vi "S4GEI.vi"() -> ()   [LabVIEW 2018]
uses:
  S4GEI/S4GEI.lvclass
  S4GEI/S4GEI.lvclass/S4GEI.ctl
  Channel GUI/Channel.lvclass/Channel.ctl
  Channel GUI/Channel.lvclass
  Camera/Camera.lvclass
  S4ICS/S4ICS.lvclass
  Mechanism/Mechanism.lvclass
panel:
  in  "Tab Control 2":T1(tab)
  in  "Stop Application":bool
  out "pol mode":bool
  out "phot mode":bool
  out "Error Message":string
  in  "wppos presents":u16(ring) items=["Clear", "All positions", "First 8 positions", "First 4 positions", "1-4 & 9-12", "Customized"]
  in  "waveplate":u16(ring)=2 items=["OFF"=2, "L/2"=3, "L/4"=1]
  in  "calib wheel":u16(ring)=3 items=["OFF"=3, "PINHOLE"=1, "POLARIZER"=2, "SHUTTER"=4, "DEPOLARIZER"=5]
  in  "waveplate positions":T2={"WP 1"=TRUE, "WP 2"=FALSE, "WP 3"=FALSE, "WP 4"=FALSE, "WP 5"=FALSE, "WP 6"=FALSE, "WP 7"=FALSE, "WP 8"=FALSE, "WP 9"=FALSE, "WP 10"=FALSE, "WP 11"=FALSE, "WP 12"=FALSE, "WP 13"=FALSE, "WP 14"=FALSE, "WP 15"=FALSE, "WP 16"=FALSE}
  out "current calw":u16(ring)=3 items=["PINHOLE"=1, "POLARIZER"=2, "OFF"=3, "SHUTTER"=4, "DEPOLARIZER"=5]
  out "current waveplate":u16(ring)=2 items=["L/4"=1, "OFF"=2, "L/2"=3]
  out "analyser status":bool
  out "current wppos":T2
  in  "start exp":bool
  in  "Stop Acquisition":bool
  in  "Abort Acquisition":bool
  in  "Pause acquisition":bool
  in  "exp time":dbl=1.5 min=9.999999747378752e-06
  in  "#frames":u16=1 min=1 max=1000
  in  "#cycles":u32=1 min=1
  in  "Send Message":bool
  in  "Command:":string
  in  "FWCS IP":string="200.131.64.49"
  in  "ACS IP":string="200.131.64.25"
  in  "Channel ID":u16=1 min=1
  out "CCD status":T3={"Cycles done"=1, "Sequences done"=1, "Frames done"=1, "CCD Status"="", "Exposing"=FALSE, "Last image"="", "temp"=0, "serial n"=0, "texp"=0.0, "used disk"=0, "power"=FALSE, "acs mode"=FALSE} {"Frames done" max=2 scale=0.0..1.0; "Sequences done" max=8 scale=0.0..1.0; "Cycles done" max=2 scale=0.0..1.0}
  in  "projid":string="ENG"
  in  "observer":string="Denis"
  in  "object name":string="Test"
  in  "comment":string
  in  "file name suffix":string
  in  "preset modes":T4
  in  "auto adv mode":bool
  in  "Cooler":bool
  in  "Temp":i32=20 min=-80 max=20
  in  "Set camera configuration":bool
  in  "EM Gain":u16=2
  in  "EM Mode":u8(ring)=1 items=["Electron Multiplying", "Conventional", "Error"]
  in  "Readout Rate":u8(ring) items=["1 MHz", "0.1 MHz"]
  in  "Pre-amp gain":u8(ring) items=["Gain 1", "Gain 2", "Error"]
  in  "Vertical Clock Voltagem":u16(ring) items=["Normal", "+1", "+2", "+3", "+4", "Error"]
  in  "Acquisition Mode":u16(ring)=3 items=["Reserved", "Single Scan", "Accumulate", "Kinetic", "Fast Kinetic", "Run till abort", "Reserved", "Reserved", "Reserved", "Time Delayed Integration"]
  in  "Read Mode":u16(ring)=4 items=["Full Vertical Binning", "Multi-Track", "Random-Track", "Single-Track", "Image"]
  in  "Trigger Mode":u16(ring) items=["Internal", "External", "N/A", "N/A", "N/A", "N/A", "External Start", "External Exposure (Bulb)", "N/A", "External FVB EM", "Software", "N/A", "External Charge Shifting"]
  in  "Vertical Shift Speed":u16(ring)=3 items=["0.6", "1.13", "2.2", "4.33", "Error"]
  in  "AD Channel":u16
  in  "Shutter Mode":u8(ring)=2 items=["OPEN"=1, "CLOSED"=2, "Error"=3]
  in  "Shutter Time":u16=50
  in  "Shutter TTL":u16(ring) items=["TTL Low", "TTL High", "Error"]
  in  "Binning":u16=1
  in  "Initial Line":u16=1
  in  "Initial Cloumn":u16=1
  in  "Final Column":u16=1024
  in  "Final Line":u16=1024
  in  "Sub Image":T5(radio)=enum."1024 x 1024"
  in  "Frame Tansfer":bool=TRUE
  in  "stop iterations":bool
  out "Exposing 2":bool
  out "Frame exp time (s) \n2":dbl
  out "Exposições realizadas 2":u16(slide)=1 max=2 scale=-1.0..1.0
  in  "Acquisition configuration 6":T6={"Select"=FALSE, "Exp Time"=1.0, "#Frames"=1, "Sufix"="", "Filter"=6} {"Filter" items=["U"=1, "B"=2, "V"=3, "R"=4, "I"=5, "Clear"=6]}
  in  "Acquisition configuration 5":T6={"Select"=FALSE, "Exp Time"=1.0, "#Frames"=1, "Sufix"="", "Filter"=5} {"Filter" items=["U"=1, "B"=2, "V"=3, "R"=4, "I"=5, "Clear"=6]}
  in  "Acquisition configuration 4":T6={"Select"=FALSE, "Exp Time"=1.0, "#Frames"=1, "Sufix"="", "Filter"=4} {"Filter" items=["U"=1, "B"=2, "V"=3, "R"=4, "I"=5, "Clear"=6]}
  in  "Acquisition configuration 3":T6={"Select"=FALSE, "Exp Time"=1.0, "#Frames"=1, "Sufix"="", "Filter"=3} {"Filter" items=["U"=1, "B"=2, "V"=3, "R"=4, "I"=5, "Clear"=6]}
  in  "Acquisition configuration 2":T6={"Select"=FALSE, "Exp Time"=1.0, "#Frames"=1, "Sufix"="", "Filter"=2} {"Filter" items=["U"=1, "B"=2, "V"=3, "R"=4, "I"=5, "Clear"=6]}
  in  "Number of iterations":u16=1
  out "Current filter":u16(ring)=1 items=["U"=1, "B"=2, "V"=3, "R"=4, "I"=5, "Clear"=6]
  in  "Start Iterations":bool
  out "Iterations Done":u16(slide) scale=0.0..1.0
  in  "Acquisition configuration":T6={"Select"=FALSE, "Exp Time"=1.0, "#Frames"=1, "Sufix"="", "Filter"=1} {"Filter" items=["U"=1, "B"=2, "V"=3, "R"=4, "I"=5, "Clear"=6]}
  out "WPROT status":T7
  out "WPSEL status":T7
  out "CALW status":T7
  out "ASEL status":T7
  out "GMIR status":T7
  out "GFOC status":T7
  # "Instrument mode:"
  # "SPARC4\nGraphical Engineering Interface (S4GEI)"
  # "AUTOMATIC ADVANCE MODE"
  # "FWCS Iterator"
  # "Select"
  # "Filter"
  # "#Frames"
  # "Exp time (s)"
  # "Suffix"
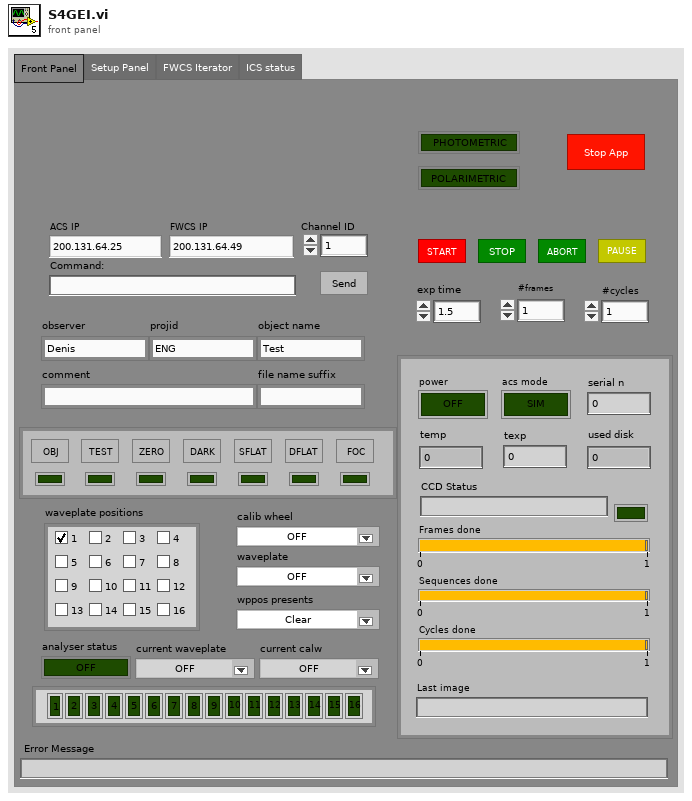
[diagram p1: front panel]
types:
  T1 = enum32{"Front Panel", "Setup Panel", "FWCS Iterator", "ICS status"}
  T2 = cluster{"WP 1":bool, "WP 2":bool, "WP 3":bool, "WP 4":bool, "WP 5":bool, "WP 6":bool, "WP 7":bool, "WP 8":bool, "WP 9":bool, "WP 10":bool, "WP 11":bool, "WP 12":bool, "WP 13":bool, "WP 14":bool, "WP 15":bool, "WP 16":bool}
  T3 = cluster{"Cycles done":u16, "Sequences done":u16, "Frames done":u16, "CCD Status":string, "Exposing":bool, "Last image":string, "temp":i16, "serial n":u16, "texp":dbl, "used disk":i16, "power":bool, "acs mode":bool}
  T4 = cluster{"OBJECT":bool, "TEST":bool, "ZERO":bool, "DARK":bool, "SFLAT":bool, "DFLAT":bool, "FOCUS":bool, "led object":bool, "led test":bool, "led zero":bool, "led dark":bool, "led sflat":bool, "led dflat":bool, "led foc":bool}
  T5 = enum32{"256 x 256", "512 x 512", "1024 x 1024", "Custom"}
  T6 = cluster{"Select":bool, "Exp Time":dbl, "#Frames":u16, "Sufix":string, "Filter":u16}
  T7 = cluster{"mode":string, "condition":string, "position":string, "pos_name":string, "pos_id":string}
  T8 = cluster{"FWCS IP":string, "ACS IP":string, "Channel ID":u16}
  T9 = enum8{"Enabled", "Disabled", "Disabled and Grayed Out"}
  T10 = cluster{"object":bool, "test":bool, "zero":bool, "dark":bool, "sflat":bool, "dflat":bool, "focus":bool, "object 2":bool, "test 2":bool, "zero 2":bool, "dark 2":bool, "sflat 2":bool, "dflat 2":bool, "foc":bool}
  T11 = cluster{"WP 1":bool, "WP 2":bool, "WP 3":bool, "WP 4":bool, "WP 5":bool, "WP 6":bool, "WP 9":bool, "WP 8":bool, "WP 7":bool, "WP 10":bool, "WP 11":bool, "WP 12":bool, "WP 13":bool, "WP 14":bool, "WP 15":bool, "WP 16":bool}
  T12 = cluster{"OBJECT":bool, "TEST":bool, "ZERO":bool, "DARK":bool, "SFLAT":bool, "DFLAT":bool, "FOCUS":bool}
  T13 = cluster{"CYCLES_DONE":u16, "LAST_IMAGE_NAME":string, "USED_DISK_SPACE":u16, "FRAMES_DONE":u16, "CCD_STATUS":string, "CURRENT_TEMPERATURE":i16, "TEMPERATURE_STATUS":string, "FRAME_EXPOSURE_TIME":sgl, "ERROR":bool, "SERIAL_NUMBER":u16, "ACQUIRING":bool, "IMAGE_INDEX":u32, "SEQS_DONE":u16, "POWER":bool, "ACS MODE":bool}
  T14 = cluster{"EXPTIME":dbl, "#FRAMES":u32, "#CYCLES":u32, "#SEQS":u32, "WAVEPLATE_POS":u16, "suffix":string, "TEMP":i32, "COOLER_POWER_STATUS":u16}
  T15 = cluster{"WPROT":refnum<class "Mechanism.lvclass">, "WPSEL":refnum<class "Mechanism.lvclass">, "CALW":refnum<class "Mechanism.lvclass">, "ASEL":refnum<class "Mechanism.lvclass">, "GMIR":refnum<class "Mechanism.lvclass">, "GFOC":refnum<class "Mechanism.lvclass">, "State Machine.lvclass":refnum<class "State Machine.lvclass">, "Status RxTx.lvclass":refnum<class "RxTx.lvclass">}
  T16 = cluster{"PREAMP":u16, "READOUT_RATE":u16, "EM_GAIN":u16, "VERTICAL_SHIFT_SPEED":u16, "READ_MODE":u16, "FRAME_TRANSFER":bool, "VERTICAL_CLOCK_VOLTAGE":u16, "ACQUISITION_MODE":u16, "AD_CHANNEL":u16, "EM_MODE":u16, "SHUTTER_TTL":u16, "SHUTTER_OPENING_TIME":u16, "SHUTTER_CLOSING_TIME":u16, "SHUTTER_MODE":u16, "TRIGGER_MODE":u16, "VBIN":u16, "INITIAL_LINE":u16, "INITIAL_COLUMN":u16, "FINAL_LINE":u16, "FINAL_COLUMN":u16, "HBIN":u16}
  T17 = cluster{"waveplate positions":cluster{"WP 1":bool, "WP 2":bool, "WP 3":bool, "WP 4":bool, "WP 5":bool, "WP 6":bool, "WP 9":bool, "WP 8":bool, "WP 7":bool, "WP 10":bool, "WP 11":bool, "WP 12":bool, "WP 13":bool, "WP 14":bool, "WP 15":bool, "WP 16":bool}, "wppos presents":u16, "calib wheel":u16, "waveplate":u16}
  T18 = cluster{"Acquire":bool, "Stop Acquisition":bool, "Abort Acquisition":bool, "Pause acquisition":bool}
  T19 = cluster{"OBJECT":string, "OBSERVER":string, "CTRLINTE":string, "PROJID":string, "SYNCMODE":string, "INSTMODE":string, "FILTER":string, "OBSTYPE":string, "GUIVRSN":string, "COMMENT":string, "broker":string, "timestamp":string, "CHANNEL 1":bool, "CHANNEL 2":bool, "CHANNEL 3":bool, "CHANNEL 4":bool, "TCSMODE":bool}
  T20 = cluster{"Cycles done":u16, "Sequences done":u16, "Frames done":u16, "CCD Status":string, "Exposing":bool, "Last image":string, "temp":i16, "serial n":u16, "texp":dbl, "used disk":i16, "Power":bool, "ACS mode":bool}
  T21 = cluster{"object":bool, "test":bool, "zero":bool, "dark":bool, "sflat":bool, "dflat":bool, "focus":bool, "led object":bool, "led test":bool, "led zero":bool, "led dark":bool, "led sflat":bool, "led dflat":bool, "led foc":bool}
  T22 = cluster{"Select":bool, "Exp Time":u16, "#Frames":u16, "Sufix":string, "Filter":u16}
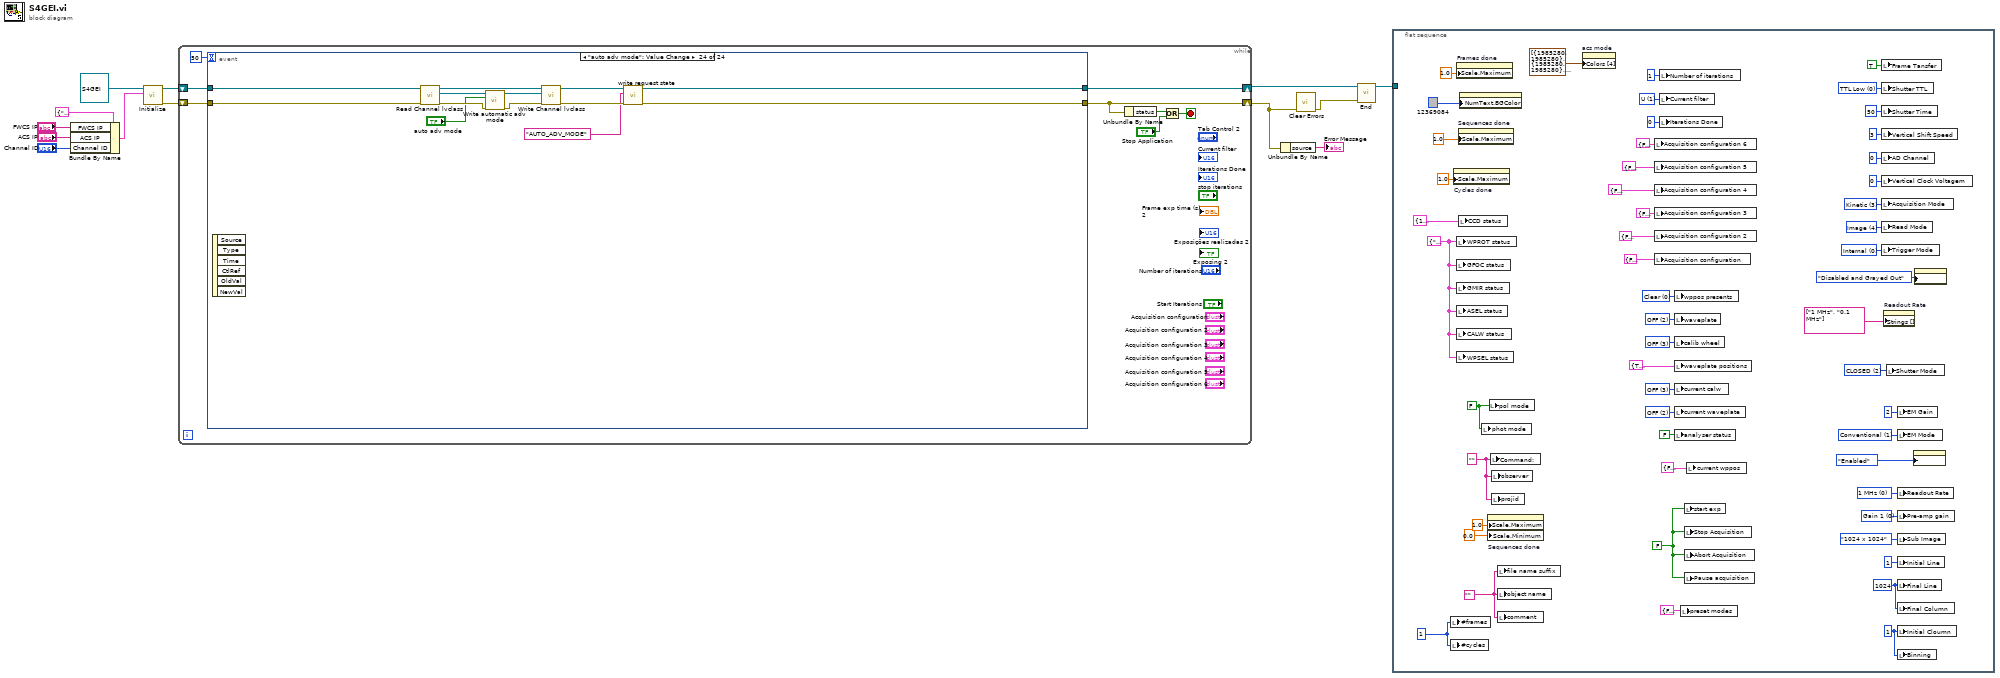
[diagram p0: block diagram]
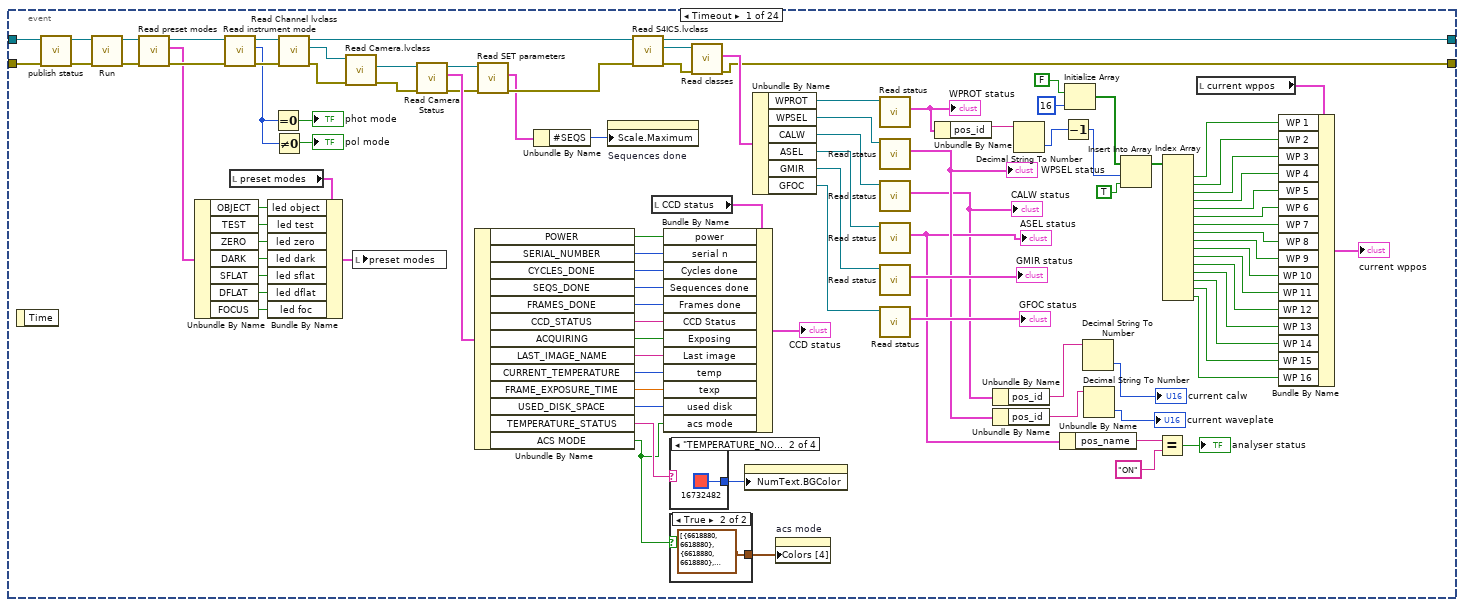
[diagram p2: hidden frame]
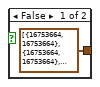
[diagram p3: hidden frame]
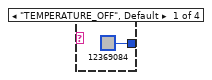
[diagram p4: hidden frame]
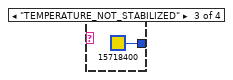
[diagram p5: hidden frame]
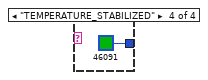
[diagram p6: hidden frame]
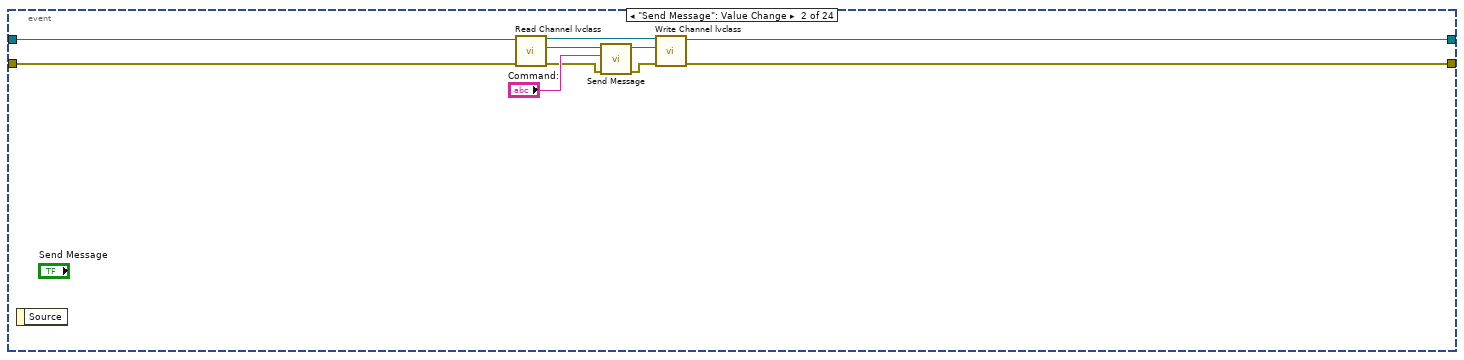
[diagram p7: hidden frame]
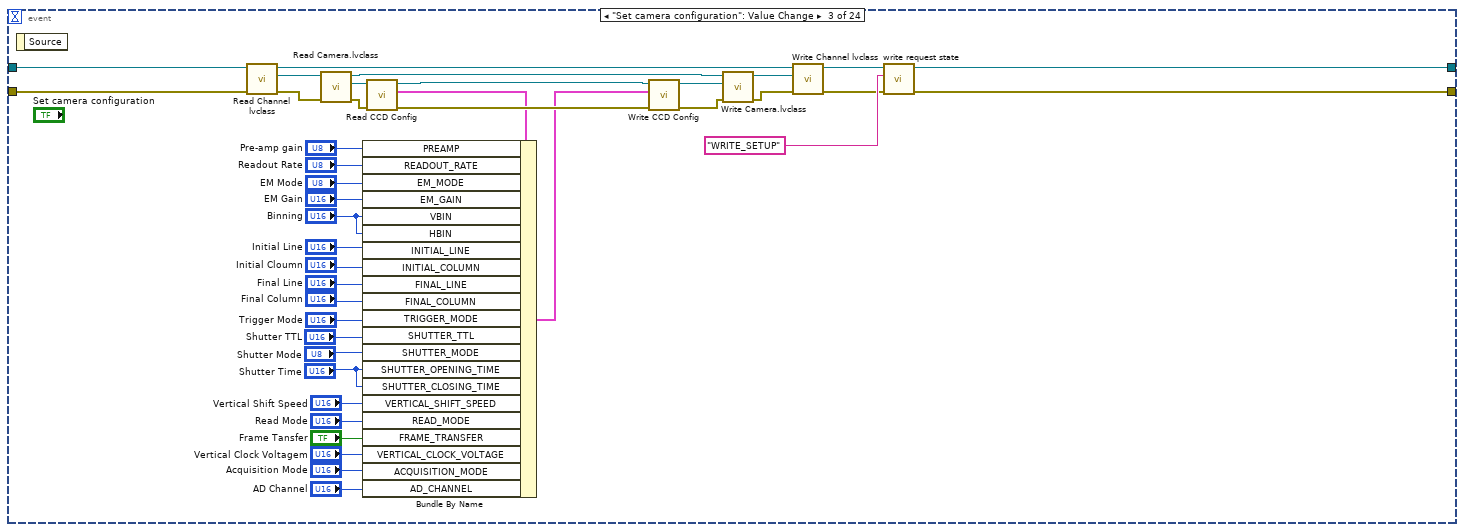
[diagram p8: hidden frame]
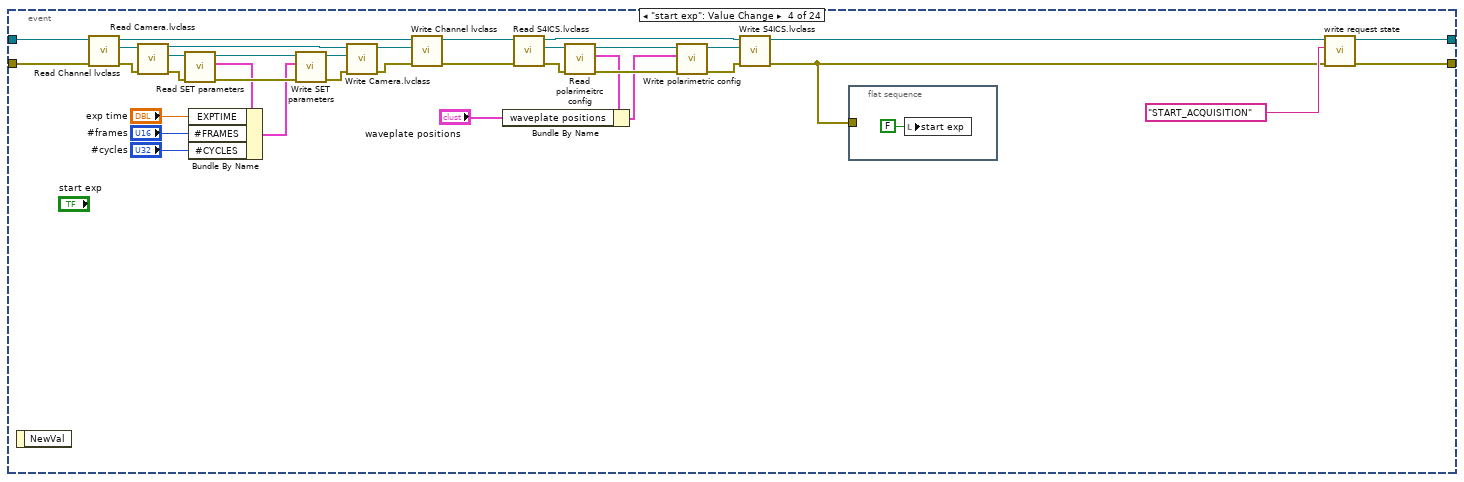
[diagram p9: hidden frame]
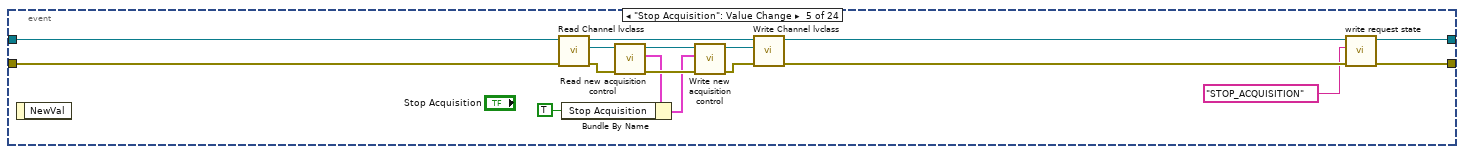
[diagram p10: hidden frame]
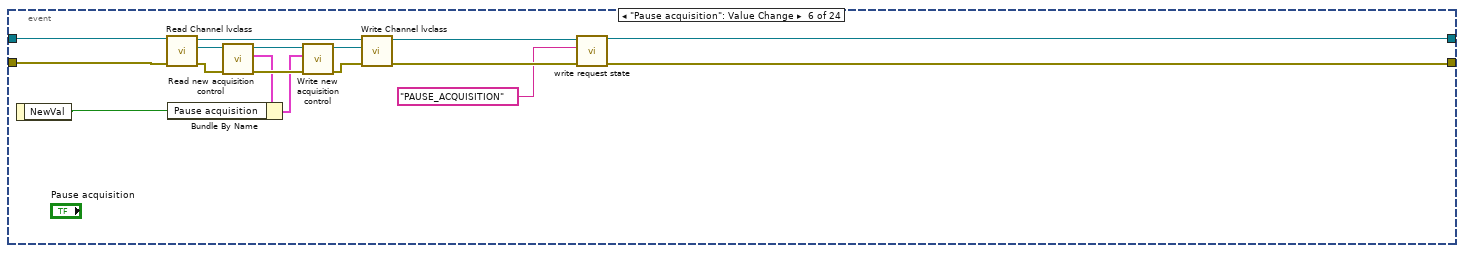
[diagram p11: hidden frame]
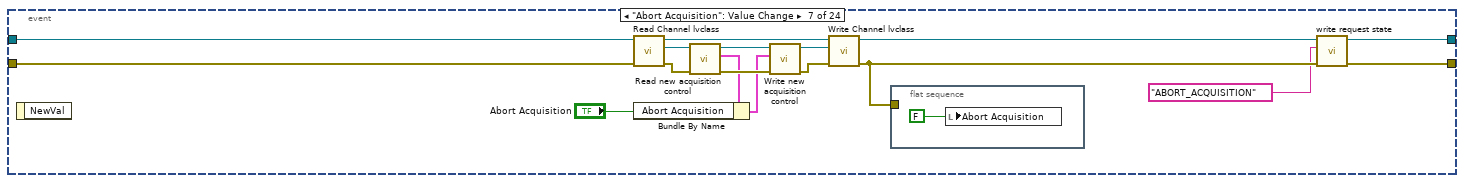
[diagram p12: hidden frame]
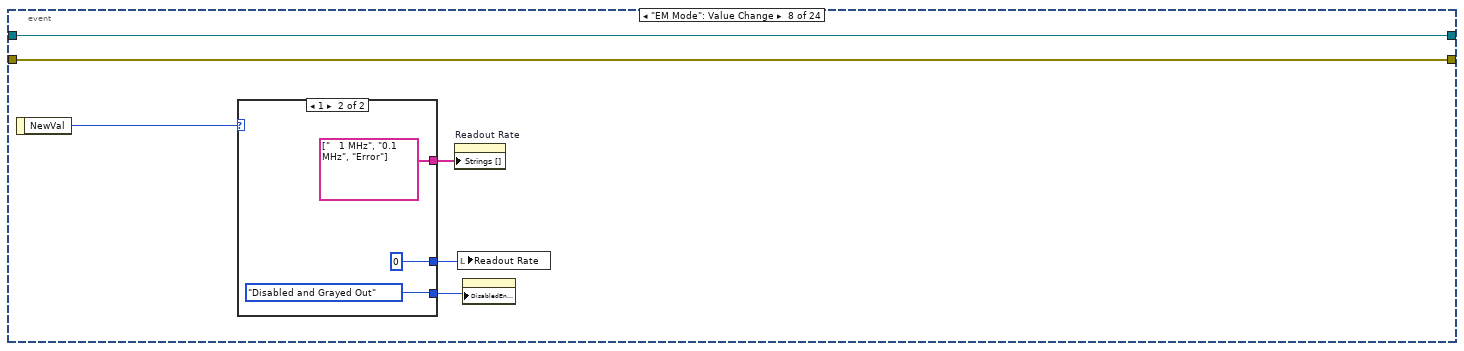
[diagram p13: hidden frame]
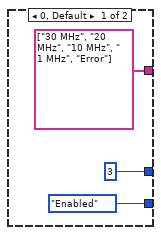
[diagram p14: hidden frame]
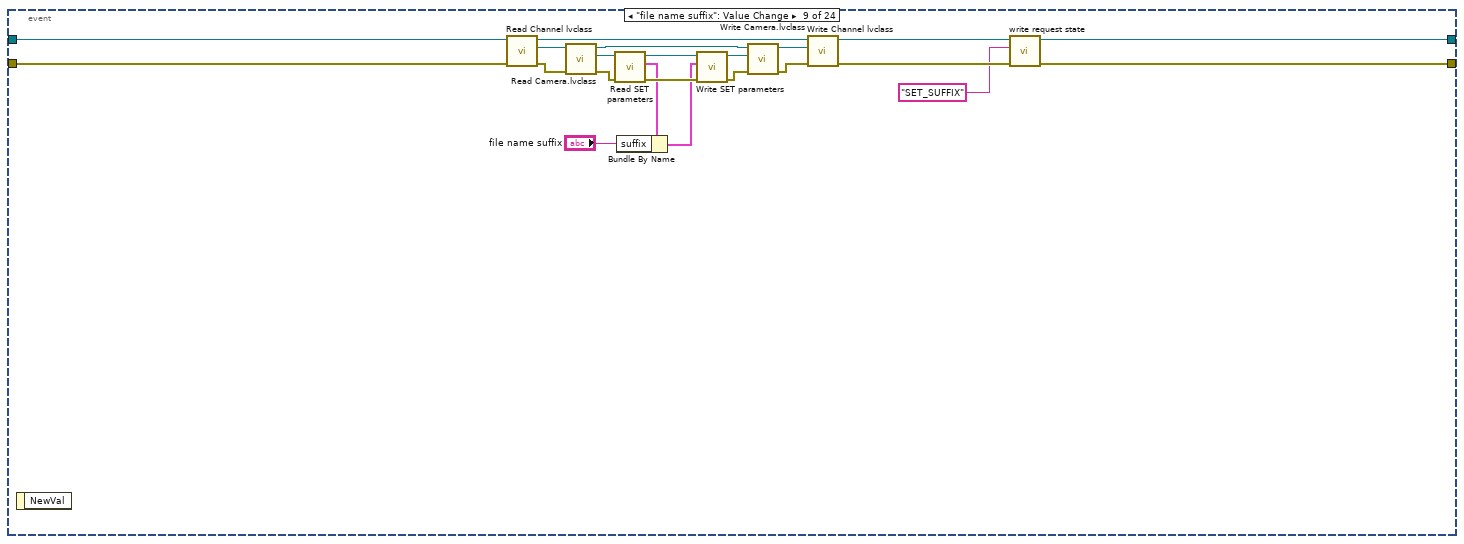
[diagram p15: hidden frame]
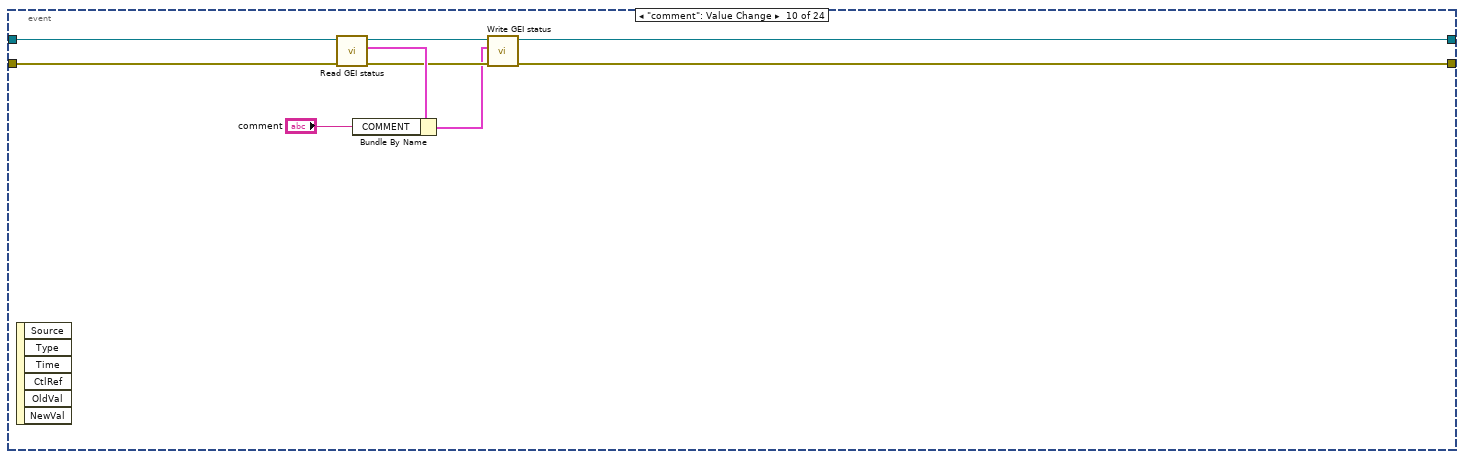
[diagram p16: hidden frame]
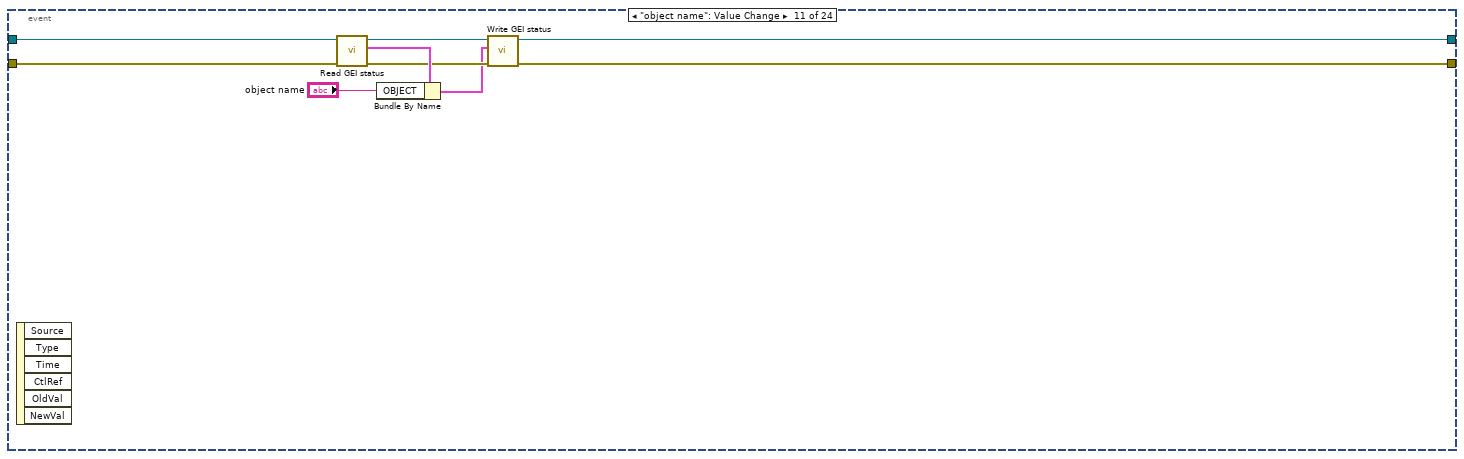
[diagram p17: hidden frame]
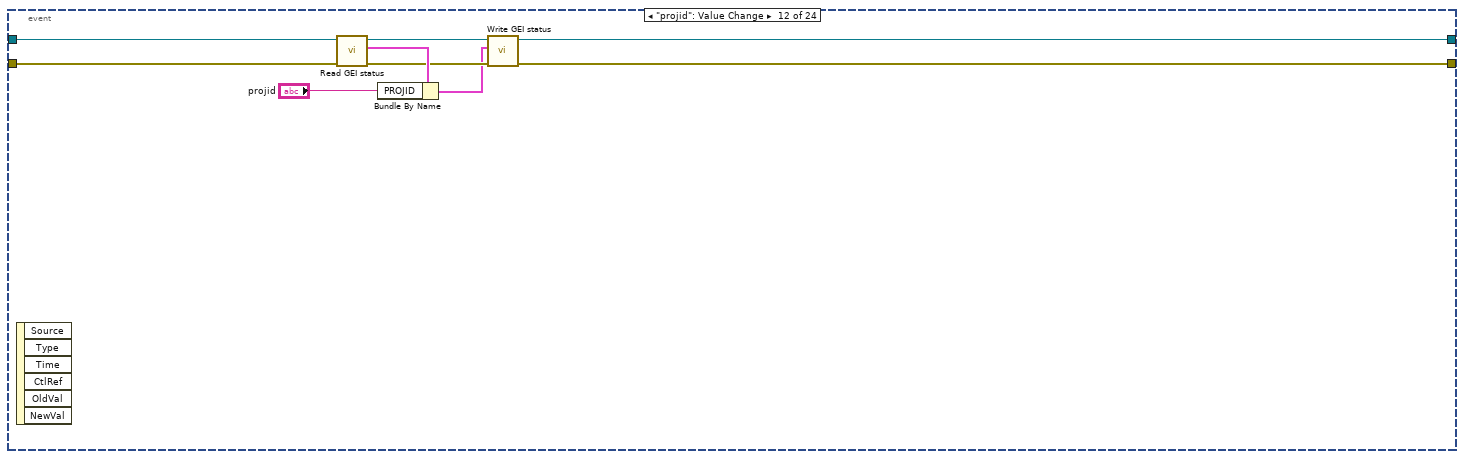
[diagram p18: hidden frame]
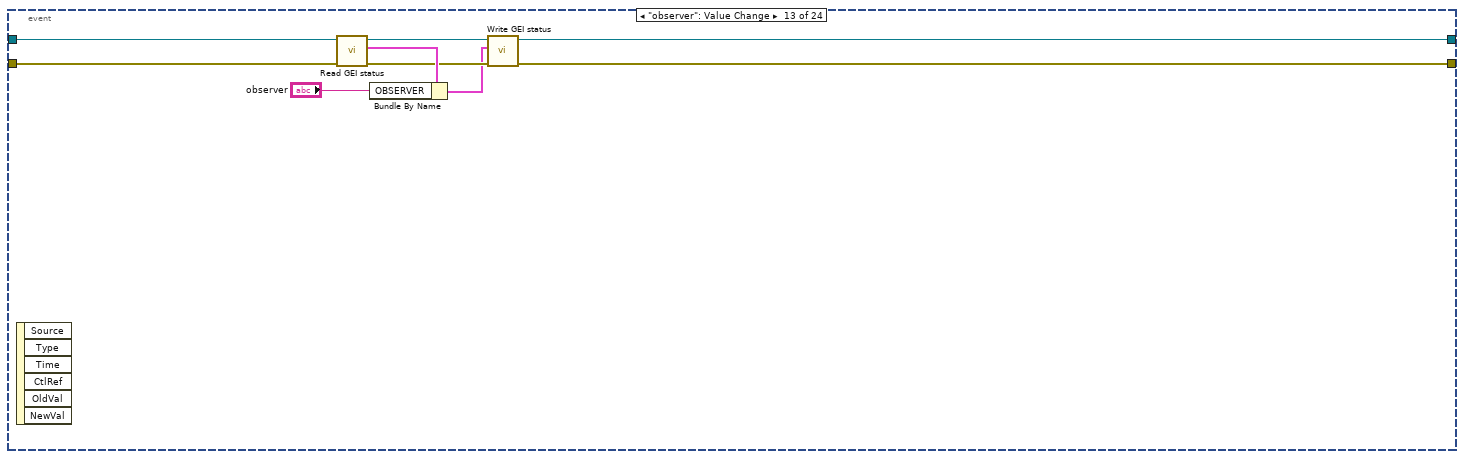
[diagram p19: hidden frame]
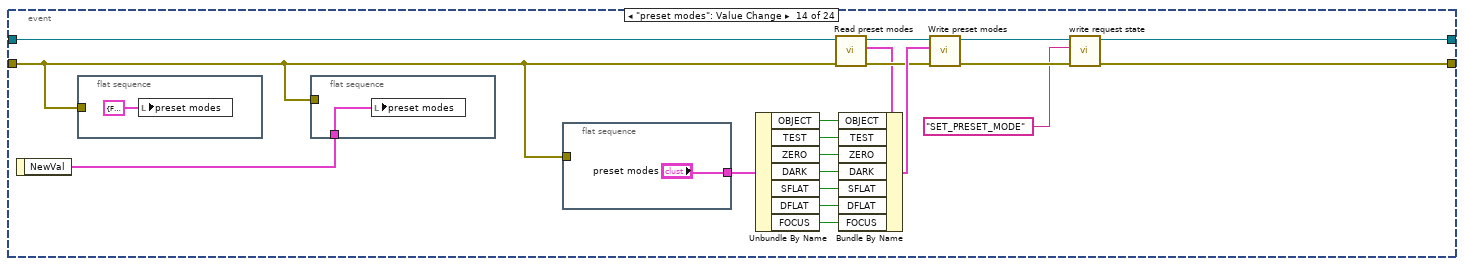
[diagram p20: hidden frame]
diagram:
  n1 = Bundle By Name(cluster=T8 {"FWCS IP"="200.131.64.49", "ACS IP"="200.131.64.25", "Channel ID"=1} ("Communication variables"), "FWCS IP"="FWCS IP", "ACS IP"="ACS IP", "Channel ID"="Channel ID") -> (w7:T8)
  n2 = call "Initialize.vi"("Communication variables"=w7, "SPARC4_GUI in"=refnum<class "S4GEI.lvclass"> refnum ("SPARC4_GUI.lvclass")) -> ("error out"=w2:errorcluster, "SPARC4_GUI out"=w1:refnum<class "S4GEI.lvclass">)  [unwired: 8 in]
  n3 = while {
    shift-right: [w14] -> w10
    shift-left: w2 -> [w16]
    shift-right: [w15] -> w12
    shift-left: w1 -> [w17]
    stop <- w20 stop-if-true
    n4 = event shown="[23] \"auto adv mode\": Value Change" {
      selector: _ -> [_ _ _ _ _ _ _ _ _ _ _ _ _ _ _ _ _ _ _ _ _ _ _ _]
      dyn-events: _ -> [_ _ _ _ _ _ _ _ _ _ _ _ _ _ _ _ _ _ _ _ _ _ _ _]
      timeout: 50 -> [_ _ _ _ _ _ _ _ _ _ _ _ _ _ _ _ _ _ _ _ _ _ _ _]
      tunnel: w16 -> [w119 w136 w177 w212 w230 w239 w256 w272 w300 w307 w316 w325 w334 w347 w362 w365 w383 w406 w424 w443 w452 w474 w496 w513]
      tunnel: [w37 w129 w140 w197 w220 w235 w251 w272 w281 w308 w317 w326 w335 w354 w362 w365 w381 w406 w411 w428 w452 w460 w484 w515] -> w14
      tunnel: w17 -> [w120 w137 w178 w213 w231 w240 w257 w273 w299 w309 w318 w327 w336 w346 w363 w366 w384 w405 w425 w444 w451 w475 w497 w514]
      tunnel: [w96 w130 w139 w198 w221 w234 w252 w273 w282 w310 w319 w328 w337 w353 w363 w366 w382 w405 w412 w427 w451 w461 w485 w516] -> w15
      event Timeout {
        n5 = event-data() -> ()  [unwired: 1 in, 1 out]
        n6 = call "publish status.vi"("error in (no error)"=w119, "S4GEI in"=w120) -> ("error out"=w118:errorcluster, "S4GEI out"=w117:refnum<class "S4GEI.lvclass">)  [unwired: 8 in]
        n7 = call "Run.vi"("error in (no error)"=w118, "SPARC4_GUI in"=w117) -> ("error out"=w48:errorcluster, "SPARC4_GUI out"=w51:refnum<class "S4GEI.lvclass">)  [unwired: 8 in]
        n8 = call-dynamic "Read preset modes.vi"("error in (no error)"=w48, "S4GEI in"=w51) -> ("error out"=w49:errorcluster, "preset modes"=w45:T12, "S4GEI out"=w50:refnum<class "S4GEI.lvclass">)  [unwired: 7 in]
        n9 = Unbundle By Name(w45) -> ("OBJECT"=w38:bool, "TEST"=w39:bool, "ZERO"=w40:bool, "DARK"=w41:bool, "SFLAT"=w42:bool, "DFLAT"=w43:bool, "FOCUS"=w44:bool)
        n10 = call-dynamic "Read instrument mode.vi"("error in (no error)"=w49, "S4GEI in"=w50) -> ("error out"=w88:errorcluster, "instrument mode"=w86:u16, "S4GEI out"=w89:refnum<class "S4GEI.lvclass">)  [unwired: 7 in]
        n11 = local read "preset modes"() -> (w47:T4)
        n12 = Bundle By Name(cluster=w47, "led object"=w38, "led test"=w39, "led zero"=w40, "led dark"=w41, "led sflat"=w42, "led dflat"=w43, "led foc"=w44) -> (w46:T4)
        n13 = Equal To 0?(x=w86) -> (x = 0?=→"phot mode":bool)
        n14 = Not Equal To 0?(x=w86) -> (x != 0?=→"pol mode":bool)
        n15 = call "Read Channel lvclass.vi"("error in (no error)"=w88, "SPARC4_GUI in"=w89) -> ("error out"=w114:errorcluster, "Channel.lvclass"=w116:refnum<class "Channel.lvclass">, "SPARC4_GUI out"=w100:refnum<class "S4GEI.lvclass">)  [unwired: 7 in]
        n16 = call-dynamic "Read Camera.lvclass.vi"("error in (no error)"=w114, "Channel in"=w116) -> ("error out"=w113:errorcluster, "Camera.lvclass"=w115:refnum<class "Camera.lvclass">)  [unwired: 7 in, 1 out]
        n17 = local write "preset modes"(w46) -> ()
        n18 = call-dynamic "Read Camera Status.vi"("error in (no error)"=w113, "Camera in"=w115) -> ("error out"=w85:errorcluster, "Camera Status"=w121:T13, "Camera out"=w84:refnum<class "Camera.lvclass">)  [unwired: 7 in]
        n19 = Unbundle By Name(w121) -> ("POWER"=w24:bool, "SERIAL_NUMBER"=w25:u16, "CYCLES_DONE"=w110:u16, "SEQS_DONE"=w109:u16, "FRAMES_DONE"=w108:u16, "CCD_STATUS"=w107:string, "ACQUIRING"=w106:bool, "LAST_IMAGE_NAME"=w105:string, "CURRENT_TEMPERATURE"=w104:i16, "FRAME_EXPOSURE_TIME"=w103:sgl, "USED_DISK_SPACE"=w102:u16, "TEMPERATURE_STATUS"=w101:string, "ACS MODE"=w22:bool)
        n20 = call-dynamic "Read SET parameters.vi"("error in (no error)"=w85, "Camera in"=w84) -> ("error out"=w83:errorcluster, "SET parameters"=w82:T14)  [unwired: 7 in, 1 out]
        n21 = Unbundle By Name(w82) -> ("#SEQS"=w81:u32)
        n22 = property on="Sequences done" class="Slide (strict)"("Scale.Maximum"=w81) -> ()  [unwired: 2 in, 2 out]
        n23 = call-dynamic "Read S4ICS.lvclass.vi"("error in (no error)"=w83, "S4GEI in"=w100) -> ("error out"=w98:errorcluster, "S4ICS.lvclass"=w99:refnum<class "S4ICS.lvclass">, "S4GEI out"=w96:refnum<class "S4GEI.lvclass">)  [unwired: 7 in]
        n24 = local read "CCD status"() -> (w112:T3)
        n25 = Bundle By Name(cluster=w112, "power"=w24, "serial n"=w25, "Cycles done"=w110, "Sequences done"=w109, "Frames done"=w108, "CCD Status"=w107, "Exposing"=w106, "Last image"=w105, "temp"=w104, "texp"=w103, "used disk"=w102, "acs mode"=w22) -> (→"CCD status":T3)
        n26 = case shown="\"TEMPERATURE_NOT_REACHED\"" w101 {
          tunnel: [u32 12369084 u32 16732482 u32 15718400 u32 46091] -> w122
          frame "TEMPERATURE_OFF", Default {
          }
          frame "TEMPERATURE_NOT_REACHED" {
          }
          frame "TEMPERATURE_NOT_STABILIZED" {
          }
          frame "TEMPERATURE_STABILIZED" {
          }
        }
        n27 = case shown="True" w22 {
          tunnel: [cluster{u32, u32}[] [{16753664, 16753664}, {16753664, 16753664}, {16753664, 16753664}] ("Colors [4]") cluster{u32, u32}[] [{6618880, 6618880}, {6618880, 6618880}, {6618880, 6618880}] ("Colors [4]")] -> w23
          frame False {
          }
          frame True {
          }
        }
        n28 = call-dynamic "Read classes.vi"("error in (no error)"=w98, "S4ICS in"=w99) -> ("error out"=w37:errorcluster, "mechanism"=w97:T15)  [unwired: 7 in, 1 out]
        n29 = property on="temp" class="DigNum (strict)"("NumText.BGColor"=w122) -> ()  [unwired: 2 in, 2 out]
        n30 = Unbundle By Name(w97) -> ("WPROT"=w95:refnum<class "Mechanism.lvclass">, "WPSEL"=w94:refnum<class "Mechanism.lvclass">, "CALW"=w93:refnum<class "Mechanism.lvclass">, "ASEL"=w92:refnum<class "Mechanism.lvclass">, "GMIR"=w91:refnum<class "Mechanism.lvclass">, "GFOC"=w90:refnum<class "Mechanism.lvclass">)
        n31 = property on="acs mode" class="Bool (strict)"("Colors [4]"=w23) -> ()  [unwired: 2 in, 2 out]
        n32 = call-dynamic "Read status.vi"("Mechanism in"=w95) -> ("status"=w79:T7)  [unwired: 8 in, 2 out]
        "WPROT status" <- w79
        n33 = call-dynamic "Read status.vi"("Mechanism in"=w94) -> ("status"=w33:T7)  [unwired: 8 in, 2 out]
        "WPSEL status" <- w33
        n34 = call-dynamic "Read status.vi"("Mechanism in"=w93) -> ("status"=w31:T7)  [unwired: 8 in, 2 out]
        "CALW status" <- w31
        n35 = call-dynamic "Read status.vi"("Mechanism in"=w92) -> ("status"=w32:T7)  [unwired: 8 in, 2 out]
        "ASEL status" <- w32
        n36 = call-dynamic "Read status.vi"("Mechanism in"=w91) -> ("status"=→"GMIR status":T7)  [unwired: 8 in, 2 out]
        n37 = call-dynamic "Read status.vi"("Mechanism in"=w90) -> ("status"=→"GFOC status":T7)  [unwired: 8 in, 2 out]
        n38 = Unbundle By Name(w79) -> ("pos_id"=w36:string)
        n39 = Unbundle By Name(w31) -> ("pos_id"=w28:string)
        n40 = Unbundle By Name(w33) -> ("pos_id"=w30:string)
        n41 = Decimal String To Number(string=w36) -> (number=w26:i32)  [unwired: 2 in, 1 out]
        n42 = Unbundle By Name(w32) -> ("pos_name"=w62:string)
        n43 = Decrement(x=w26) -> (x-1=w58:i32)
        n44 = Initialize Array(FALSE, 16 ("dimension size")) -> (w55:bool[])
        n45 = Decimal String To Number(string=w28) -> (number=→"current calw":i32)  [unwired: 2 in, 1 out]
        n46 = Decimal String To Number(string=w30) -> (number=→"current waveplate":i32)  [unwired: 2 in, 1 out]
        n47 = Insert Into Array(array=w55, index=w58, new element=TRUE ("new element/subarray")) -> (w60:bool[])
        n48 = Equal?(x=w62, y="ON") -> (x = y?=→"analyser status":bool)
        n49 = Index Array(array=w60) -> (element #1=w78:bool, element #2=w77:bool, element #3=w76:bool, element #4=w75:bool, element #5=w74:bool, element #6=w73:bool, element #7=w72:bool, element #8=w71:bool, element #9=w70:bool, element #10=w69:bool, element #11=w68:bool, element #12=w67:bool, element #13=w66:bool, element #14=w65:bool, element #15=w64:bool, element #16=w63:bool)  [unwired: 16 in]
        n50 = local read "current wppos"() -> (w54:T2)
        n51 = Bundle By Name(cluster=w54, "WP 1"=w78, "WP 2"=w77, "WP 3"=w76, "WP 4"=w75, "WP 5"=w74, "WP 6"=w73, "WP 7"=w72, "WP 8"=w71, "WP 9"=w70, "WP 10"=w69, "WP 11"=w68, "WP 12"=w67, "WP 13"=w66, "WP 14"=w65, "WP 15"=w64, "WP 16"=w63) -> (→"current wppos":T2)
      }
      event "Send Message": Value Change {
        n52 = event-data() -> ()  [unwired: 1 in, 1 out]
        n53 = call "Read Channel lvclass.vi"("error in (no error)"=w136, "SPARC4_GUI in"=w137) -> ("error out"=w132:errorcluster, "Channel.lvclass"=w135:refnum<class "Channel.lvclass">, "SPARC4_GUI out"=w131:refnum<class "S4GEI.lvclass">)  [unwired: 7 in]
        n54 = call "Send Message.vi"("error in (no error)"=w132, "Message"="Command:", "Channel GUI in"=w135) -> ("error out"=w133:errorcluster, "Channel GUI out"=w134:refnum<class "Channel.lvclass">)  [unwired: 7 in]
        n55 = call "Write Channel lvclass.vi"("error in (no error)"=w133, "Channel.lvclass"=w134, "SPARC4_GUI in"=w131) -> ("error out"=w129:errorcluster, "SPARC4_GUI out"=w130:refnum<class "S4GEI.lvclass">)  [unwired: 7 in]
      }
      event "Set camera configuration": Value Change {
        n56 = event-data() -> ()  [unwired: 1 in, 1 out]
        n57 = call "Read Channel lvclass.vi"("error in (no error)"=w177, "SPARC4_GUI in"=w178) -> ("error out"=w176:errorcluster, "Channel.lvclass"=w145:refnum<class "Channel.lvclass">, "SPARC4_GUI out"=w175:refnum<class "S4GEI.lvclass">)  [unwired: 7 in]
        n58 = call-dynamic "Read Camera.lvclass.vi"("error in (no error)"=w176, "Channel in"=w145) -> ("error out"=w174:errorcluster, "Camera.lvclass"=w173:refnum<class "Camera.lvclass">, "Channel out"=w144:refnum<class "Channel.lvclass">)  [unwired: 7 in]
        n59 = call-dynamic "Read CCD Config.vi"("error in (no error)"=w174, "Camera in"=w173) -> ("error out"=w172:errorcluster, "CCD Config"=w147:T16, "Camera out"=w152:refnum<class "Camera.lvclass">)  [unwired: 7 in]
        n60 = Bundle By Name(cluster=w147, "PREAMP"="Pre-amp gain", "READOUT_RATE"="Readout Rate", "EM_MODE"="EM Mode", "EM_GAIN"="EM Gain", "VBIN"="Binning", "HBIN"="Binning", "INITIAL_LINE"="Initial Line", "INITIAL_COLUMN"="Initial Cloumn", "FINAL_LINE"="Final Line", "FINAL_COLUMN"="Final Column", "TRIGGER_MODE"="Trigger Mode", "SHUTTER_TTL"="Shutter TTL", "SHUTTER_MODE"="Shutter Mode", "SHUTTER_OPENING_TIME"="Shutter Time", "SHUTTER_CLOSING_TIME"="Shutter Time", "VERTICAL_SHIFT_SPEED"="Vertical Shift Speed", "READ_MODE"="Read Mode", "FRAME_TRANSFER"="Frame Tansfer", "VERTICAL_CLOCK_VOLTAGE"="Vertical Clock Voltagem", "ACQUISITION_MODE"="Acquisition Mode", "AD_CHANNEL"="AD Channel") -> (w146:T16)
        n61 = call-dynamic "Write CCD Config.vi"("error in (no error)"=w172, "CCD Config"=w146, "Camera in"=w152) -> ("error out"=w150:errorcluster, "Camera out"=w151:refnum<class "Camera.lvclass">)  [unwired: 7 in]
        n62 = call-dynamic "Write Camera.lvclass.vi"("error in (no error)"=w150, "Camera.lvclass"=w151, "Channel in"=w144) -> ("error out"=w149:errorcluster, "Channel out"=w148:refnum<class "Channel.lvclass">)  [unwired: 7 in]
        n63 = call "Write Channel lvclass.vi"("error in (no error)"=w149, "Channel.lvclass"=w148, "SPARC4_GUI in"=w175) -> ("error out"=w142:errorcluster, "SPARC4_GUI out"=w141:refnum<class "S4GEI.lvclass">)  [unwired: 7 in]
        n64 = call "write request state.vi"("error in (no error)"=w142, "State"="WRITE_SETUP", "S4GEI in"=w141) -> ("error out"=w140:errorcluster, "S4GEI out"=w139:refnum<class "S4GEI.lvclass">)  [unwired: 7 in]
      }
      event "start exp": Value Change {
        n65 = event-data() -> ()  [unwired: 1 in, 1 out]
        n66 = call "Read Channel lvclass.vi"("error in (no error)"=w212, "SPARC4_GUI in"=w213) -> ("error out"=w211:errorcluster, "Channel.lvclass"=w200:refnum<class "Channel.lvclass">, "SPARC4_GUI out"=w214:refnum<class "S4GEI.lvclass">)  [unwired: 7 in]
        n67 = call-dynamic "Read Camera.lvclass.vi"("error in (no error)"=w211, "Channel in"=w200) -> ("error out"=w207:errorcluster, "Camera.lvclass"=w208:refnum<class "Camera.lvclass">, "Channel out"=w199:refnum<class "Channel.lvclass">)  [unwired: 7 in]
        n68 = call-dynamic "Read SET parameters.vi"("error in (no error)"=w207, "Camera in"=w208) -> ("error out"=w205:errorcluster, "SET parameters"=w202:T14, "Camera out"=w206:refnum<class "Camera.lvclass">)  [unwired: 7 in]
        n69 = Bundle By Name(cluster=w202, "EXPTIME"="exp time", "#FRAMES"="#frames", "#CYCLES"="#cycles") -> (w201:T14)
        n70 = call-dynamic "Write SET parameters.vi"("error in (no error)"=w205, "SET parameters"=w201, "Camera in"=w206) -> ("error out"=w203:errorcluster, "Camera out"=w204:refnum<class "Camera.lvclass">)  [unwired: 7 in]
        n71 = call-dynamic "Write Camera.lvclass.vi"("error in (no error)"=w203, "Camera.lvclass"=w204, "Channel in"=w199) -> ("error out"=w210:errorcluster, "Channel out"=w209:refnum<class "Channel.lvclass">)  [unwired: 7 in]
        n72 = call "Write Channel lvclass.vi"("error in (no error)"=w210, "Channel.lvclass"=w209, "SPARC4_GUI in"=w214) -> ("error out"=w194:errorcluster, "SPARC4_GUI out"=w195:refnum<class "S4GEI.lvclass">)  [unwired: 7 in]
        n73 = call-dynamic "Read S4ICS.lvclass.vi"("error in (no error)"=w194, "S4GEI in"=w195) -> ("error out"=w187:errorcluster, "S4ICS.lvclass"=w190:refnum<class "S4ICS.lvclass">, "S4GEI out"=w186:refnum<class "S4GEI.lvclass">)  [unwired: 7 in]
        n74 = call-dynamic "Read polarimeitrc config.vi"("error in (no error)"=w187, "S4ICS in"=w190) -> ("error out"=w188:errorcluster, "polarimeitrc config"=w185:T17, "S4ICS out"=w191:refnum<class "S4ICS.lvclass">)  [unwired: 7 in]
        n75 = Bundle By Name(cluster=w185, "waveplate positions"="waveplate positions") -> (w184:T17)
        n76 = call-dynamic "Write polarimetric config.vi"("error in (no error)"=w188, "polarimeitrc config"=w184, "S4ICS in"=w191) -> ("error out"=w189:errorcluster, "S4ICS out"=w192:refnum<class "S4ICS.lvclass">)  [unwired: 7 in]
        n77 = call-dynamic "Write S4ICS.lvclass.vi"("error in (no error)"=w189, "S4ICS.lvclass"=w192, "S4GEI in"=w186) -> ("error out"=w179:errorcluster, "S4GEI out"=w193:refnum<class "S4GEI.lvclass">)  [unwired: 7 in]
        n78 = flat-sequence {
          tunnel: w179 -> [_]
          frame #0 {
            n79 = local write "start exp"(FALSE ("start exp")) -> ()
          }
        }
        n80 = call "write request state.vi"("error in (no error)"=w179, "State"="START_ACQUISITION", "S4GEI in"=w193) -> ("error out"=w197:errorcluster, "S4GEI out"=w198:refnum<class "S4GEI.lvclass">)  [unwired: 7 in]
      }
      event "Stop Acquisition": Value Change {
        n81 = event-data() -> ()  [unwired: 1 in, 1 out]
        n82 = call "Read Channel lvclass.vi"("error in (no error)"=w230, "SPARC4_GUI in"=w231) -> ("error out"=w226:errorcluster, "Channel.lvclass"=w229:refnum<class "Channel.lvclass">, "SPARC4_GUI out"=w232:refnum<class "S4GEI.lvclass">)  [unwired: 7 in]
        n83 = call "Read new acquisition control.vi"("error in (no error)"=w226, "Channel in"=w229) -> ("error out"=w225:errorcluster, "new acquisition control"=w223:T18, "Channel out"=w228:refnum<class "Channel.lvclass">)  [unwired: 7 in]
        n84 = Bundle By Name(cluster=w223, "Stop Acquisition"=TRUE) -> (w222:T18)
        n85 = call "Write new acquisition control.vi"("error in (no error)"=w225, "new acquisition control"=w222, "Channel in"=w228) -> ("error out"=w224:errorcluster, "Channel out"=w227:refnum<class "Channel.lvclass">)  [unwired: 7 in]
        n86 = call "Write Channel lvclass.vi"("error in (no error)"=w224, "Channel.lvclass"=w227, "SPARC4_GUI in"=w232) -> ("error out"=w219:errorcluster, "SPARC4_GUI out"=w218:refnum<class "S4GEI.lvclass">)  [unwired: 7 in]
        n87 = call "write request state.vi"("error in (no error)"=w219, "State"="STOP_ACQUISITION", "S4GEI in"=w218) -> ("error out"=w220:errorcluster, "S4GEI out"=w221:refnum<class "S4GEI.lvclass">)  [unwired: 7 in]
      }
      event "Pause acquisition": Value Change {
        n88 = event-data() -> ("NewVal"=w238:bool)  [unwired: 1 in]
        n89 = call "Read Channel lvclass.vi"("error in (no error)"=w239, "SPARC4_GUI in"=w240) -> ("error out"=w245:errorcluster, "Channel.lvclass"=w248:refnum<class "Channel.lvclass">, "SPARC4_GUI out"=w249:refnum<class "S4GEI.lvclass">)  [unwired: 7 in]
        n90 = call "Read new acquisition control.vi"("error in (no error)"=w245, "Channel in"=w248) -> ("error out"=w244:errorcluster, "new acquisition control"=w242:T18, "Channel out"=w247:refnum<class "Channel.lvclass">)  [unwired: 7 in]
        n91 = Bundle By Name(cluster=w242, "Pause acquisition"=w238) -> (w241:T18)
        n92 = call "Write new acquisition control.vi"("error in (no error)"=w244, "new acquisition control"=w241, "Channel in"=w247) -> ("error out"=w243:errorcluster, "Channel out"=w246:refnum<class "Channel.lvclass">)  [unwired: 7 in]
        n93 = call "Write Channel lvclass.vi"("error in (no error)"=w243, "Channel.lvclass"=w246, "SPARC4_GUI in"=w249) -> ("error out"=w237:errorcluster, "SPARC4_GUI out"=w236:refnum<class "S4GEI.lvclass">)  [unwired: 7 in]
        n94 = call "write request state.vi"("error in (no error)"=w237, "State"="PAUSE_ACQUISITION", "S4GEI in"=w236) -> ("error out"=w235:errorcluster, "S4GEI out"=w234:refnum<class "S4GEI.lvclass">)  [unwired: 7 in]
      }
      event "Abort Acquisition": Value Change {
        n95 = event-data() -> ()  [unwired: 1 in, 1 out]
        n96 = call "Read Channel lvclass.vi"("error in (no error)"=w256, "SPARC4_GUI in"=w257) -> ("error out"=w262:errorcluster, "Channel.lvclass"=w265:refnum<class "Channel.lvclass">, "SPARC4_GUI out"=w266:refnum<class "S4GEI.lvclass">)  [unwired: 7 in]
        n97 = call "Read new acquisition control.vi"("error in (no error)"=w262, "Channel in"=w265) -> ("error out"=w261:errorcluster, "new acquisition control"=w259:T18, "Channel out"=w264:refnum<class "Channel.lvclass">)  [unwired: 7 in]
        n98 = Bundle By Name(cluster=w259, "Abort Acquisition"="Abort Acquisition") -> (w258:T18)
        n99 = call "Write new acquisition control.vi"("error in (no error)"=w261, "new acquisition control"=w258, "Channel in"=w264) -> ("error out"=w260:errorcluster, "Channel out"=w263:refnum<class "Channel.lvclass">)  [unwired: 7 in]
        n100 = call "Write Channel lvclass.vi"("error in (no error)"=w260, "Channel.lvclass"=w263, "SPARC4_GUI in"=w266) -> ("error out"=w253:errorcluster, "SPARC4_GUI out"=w254:refnum<class "S4GEI.lvclass">)  [unwired: 7 in]
        n101 = flat-sequence {
          tunnel: w253 -> [_]
          frame #0 {
            n102 = local write "Abort Acquisition"(FALSE ("Abort Acquisition")) -> ()
          }
        }
        n103 = call "write request state.vi"("error in (no error)"=w253, "State"="ABORT_ACQUISITION", "S4GEI in"=w254) -> ("error out"=w251:errorcluster, "S4GEI out"=w252:refnum<class "S4GEI.lvclass">)  [unwired: 7 in]
      }
      event "EM Mode": Value Change {
        n104 = event-data() -> ("NewVal"=w270:u8)  [unwired: 1 in]
        n105 = case shown="1" w270 {
          tunnel: [string[] ["30 MHz", "20 MHz", "10 MHz", "  1 MHz", "Error"] string[] ["   1 MHz", "0.1 MHz", "Error"]] -> w271
          tunnel: [3 0] -> w269
          tunnel: [T9."Enabled" ("Disabled") T9."Disabled and Grayed Out" ("Disabled")] -> w268
          frame 0, Default {
          }
          frame 1 {
          }
        }
        n106 = property on="Readout Rate" class="Ring (strict)"("Strings []"=w271) -> ()  [unwired: 2 in, 2 out]
        n107 = local write "Readout Rate"(w269) -> ()
        n108 = property on="EM Gain" class="DigNum (strict)"("DisabledEnum"=w268) -> ()  [unwired: 2 in, 2 out]
      }
      event "file name suffix": Value Change {
        n109 = event-data() -> ()  [unwired: 1 in, 1 out]
        n110 = call "Read Channel lvclass.vi"("error in (no error)"=w300, "SPARC4_GUI in"=w299) -> ("error out"=w298:errorcluster, "Channel.lvclass"=w289:refnum<class "Channel.lvclass">, "SPARC4_GUI out"=w301:refnum<class "S4GEI.lvclass">)  [unwired: 7 in]
        n111 = call-dynamic "Read Camera.lvclass.vi"("error in (no error)"=w298, "Channel in"=w289) -> ("error out"=w294:errorcluster, "Camera.lvclass"=w295:refnum<class "Camera.lvclass">, "Channel out"=w288:refnum<class "Channel.lvclass">)  [unwired: 7 in]
        n112 = call-dynamic "Read SET parameters.vi"("error in (no error)"=w294, "Camera in"=w295) -> ("error out"=w293:errorcluster, "SET parameters"=w287:T14, "Camera out"=w292:refnum<class "Camera.lvclass">)  [unwired: 7 in]
        n113 = Bundle By Name(cluster=w287, "suffix"="file name suffix") -> (w286:T14)
        n114 = call-dynamic "Write SET parameters.vi"("error in (no error)"=w293, "SET parameters"=w286, "Camera in"=w292) -> ("error out"=w296:errorcluster, "Camera out"=w297:refnum<class "Camera.lvclass">)  [unwired: 7 in]
        n115 = call-dynamic "Write Camera.lvclass.vi"("error in (no error)"=w296, "Camera.lvclass"=w297, "Channel in"=w288) -> ("error out"=w290:errorcluster, "Channel out"=w291:refnum<class "Channel.lvclass">)  [unwired: 7 in]
        n116 = call "Write Channel lvclass.vi"("error in (no error)"=w290, "Channel.lvclass"=w291, "SPARC4_GUI in"=w301) -> ("error out"=w283:errorcluster, "SPARC4_GUI out"=w284:refnum<class "S4GEI.lvclass">)  [unwired: 7 in]
        n117 = call "write request state.vi"("error in (no error)"=w283, "State"="SET_SUFFIX" ("Message"), "S4GEI in"=w284) -> ("error out"=w281:errorcluster, "S4GEI out"=w282:refnum<class "S4GEI.lvclass">)  [unwired: 7 in]
      }
      event "comment": Value Change {
        n118 = event-data() -> ()  [unwired: 1 in, 6 out]
        n119 = call-dynamic "Read GEI status.vi"("error in (no error)"=w307, "S4GEI in"=w309) -> ("error out"=w305:errorcluster, "GEI status"=w306:T19, "S4GEI out"=w304:refnum<class "S4GEI.lvclass">)  [unwired: 7 in]
        n120 = Bundle By Name(cluster=w306, "COMMENT"="comment") -> (w303:T19)
        n121 = call-dynamic "Write GEI status.vi"("error in (no error)"=w305, "GEI status"=w303, "S4GEI in"=w304) -> ("error out"=w308:errorcluster, "S4GEI out"=w310:refnum<class "S4GEI.lvclass">)  [unwired: 7 in]
      }
      event "object name": Value Change {
        n122 = event-data() -> ()  [unwired: 1 in, 6 out]
        n123 = call-dynamic "Read GEI status.vi"("error in (no error)"=w316, "S4GEI in"=w318) -> ("error out"=w314:errorcluster, "GEI status"=w315:T19, "S4GEI out"=w313:refnum<class "S4GEI.lvclass">)  [unwired: 7 in]
        n124 = Bundle By Name(cluster=w315, "OBJECT"="object name") -> (w312:T19)
        n125 = call-dynamic "Write GEI status.vi"("error in (no error)"=w314, "GEI status"=w312, "S4GEI in"=w313) -> ("error out"=w317:errorcluster, "S4GEI out"=w319:refnum<class "S4GEI.lvclass">)  [unwired: 7 in]
      }
      event "projid": Value Change {
        n126 = event-data() -> ()  [unwired: 1 in, 6 out]
        n127 = call-dynamic "Read GEI status.vi"("error in (no error)"=w325, "S4GEI in"=w327) -> ("error out"=w323:errorcluster, "GEI status"=w324:T19, "S4GEI out"=w322:refnum<class "S4GEI.lvclass">)  [unwired: 7 in]
        n128 = Bundle By Name(cluster=w324, "PROJID"="projid") -> (w321:T19)
        n129 = call-dynamic "Write GEI status.vi"("error in (no error)"=w323, "GEI status"=w321, "S4GEI in"=w322) -> ("error out"=w326:errorcluster, "S4GEI out"=w328:refnum<class "S4GEI.lvclass">)  [unwired: 7 in]
      }
      event "observer": Value Change {
        n130 = event-data() -> ()  [unwired: 1 in, 6 out]
        n131 = call-dynamic "Read GEI status.vi"("error in (no error)"=w334, "S4GEI in"=w336) -> ("error out"=w332:errorcluster, "GEI status"=w333:T19, "S4GEI out"=w331:refnum<class "S4GEI.lvclass">)  [unwired: 7 in]
        n132 = Bundle By Name(cluster=w333, "OBSERVER"="observer") -> (w330:T19)
        n133 = call-dynamic "Write GEI status.vi"("error in (no error)"=w332, "GEI status"=w330, "S4GEI in"=w331) -> ("error out"=w335:errorcluster, "S4GEI out"=w337:refnum<class "S4GEI.lvclass">)  [unwired: 7 in]
      }
      event "preset modes": Value Change {
        n134 = event-data() -> ("NewVal"=w357:T4)  [unwired: 1 in]
        n135 = flat-sequence {
          tunnel: w347 -> [_]
          frame #0 {
            n136 = local write "preset modes"(T10 {"object"=FALSE, "test"=FALSE, "zero"=FALSE, "dark"=FALSE, "sflat"=FALSE, "dflat"=FALSE, "focus"=FALSE, "object 2"=FALSE, "test 2"=FALSE, "zero 2"=FALSE, "dark 2"=FALSE, "sflat 2"=FALSE, "dflat 2"=FALSE, "foc"=FALSE} ("preset modes")) -> ()
          }
        }
        n137 = flat-sequence {
          tunnel: w347 -> [_]
          tunnel: w357 -> [w359]
          frame #0 {
            n138 = local write "preset modes"(w359) -> ()
          }
        }
        n139 = flat-sequence {
          tunnel: w347 -> [_]
          tunnel: ["preset modes"] -> w345
          frame #0 {
          }
        }
        n140 = Unbundle By Name(w345) -> ("OBJECT"=w344:bool, "TEST"=w343:bool, "ZERO"=w342:bool, "DARK"=w341:bool, "SFLAT"=w340:bool, "DFLAT"=w339:bool, "FOCUS"=w338:bool)
        n141 = call-dynamic "Read preset modes.vi"("error in (no error)"=w347, "S4GEI in"=w346) -> ("error out"=w349:errorcluster, "preset modes"=w348:T12, "S4GEI out"=w350:refnum<class "S4GEI.lvclass">)  [unwired: 7 in]
        n142 = Bundle By Name(cluster=w348, "OBJECT"=w344, "TEST"=w343, "ZERO"=w342, "DARK"=w341, "SFLAT"=w340, "DFLAT"=w339, "FOCUS"=w338) -> (w351:T12)
        n143 = call-dynamic "Write preset modes.vi"("error in (no error)"=w349, "preset modes"=w351, "S4GEI in"=w350) -> ("error out"=w355:errorcluster, "S4GEI out"=w356:refnum<class "S4GEI.lvclass">)  [unwired: 7 in]
        n144 = call "write request state.vi"("error in (no error)"=w355, "State"="SET_PRESET_MODE", "S4GEI in"=w356) -> ("error out"=w354:errorcluster, "S4GEI out"=w353:refnum<class "S4GEI.lvclass">)  [unwired: 7 in]
      }
      event "#cycles": Value Change {
        n145 = event-data() -> ("NewVal"=w361:u32)  [unwired: 1 in]
        n146 = property on="Cycles done" class="Slide (strict)"("Scale.Maximum"=w361) -> ()  [unwired: 2 in, 2 out]
      }
      event "#frames": Value Change {
        n147 = event-data() -> ("NewVal"=w364:u16)  [unwired: 1 in]
        n148 = property on="Frames done" class="Slide (strict)"("Scale.Maximum"=w364) -> ()  [unwired: 2 in, 2 out]
      }
      event "Sub Image": Value Change {
        w371 = 1024
        n149 = event-data() -> ()  [unwired: 1 in, 1 out]
        n150 = case shown="\"256 x 256\"" "Sub Image" {
          tunnel: [128 256 512 512] -> w375
          frame "256 x 256" {
          }
          frame "512 x 512" {
          }
          frame "1024 x 1024", Default {
          }
          frame "Custom" {
          }
        }
        n151 = case shown="\"Custom\"" "Sub Image" {
          tunnel: [T9."Disabled and Grayed Out" ("Disabled") T9."Enabled" ("Disabled")] -> w378
          frame "1024 x 1024", Default {
          }
          frame "Custom" {
          }
        }
        n152 = Divide(x=w371, y=2) -> (x/y=w374:dbl)
        n153 = Divide(x=w371, y=2) -> (x/y=w373:dbl)
        n154 = Add(x=w374, y=w375) -> (x+y=w367:dbl)
        n155 = Subtract(x=w374, y=w375) -> (x-y=w376:dbl)
        n156 = Subtract(x=w373, y=w375) -> (x-y=w377:dbl)
        n157 = Add(x=w373, y=w375) -> (x+y=w380:dbl)
        n158 = Increment(x=w376) -> (x+1=w379:dbl)
        n159 = Increment(x=w377) -> (x+1=w368:dbl)
        n160 = local write "Initial Cloumn"(w379) -> ()
        n161 = local write "Final Column"(w380) -> ()
        n162 = local write "Initial Line"(w368) -> ()
        n163 = local write "Final Line"(w367) -> ()
        n164 = property on="Initial Line" class="DigNum (strict)"("DisabledEnum"=w378) -> ()  [unwired: 2 in, 2 out]
        n165 = property on="Initial Cloumn" class="DigNum (strict)"("DisabledEnum"=w378) -> ()  [unwired: 2 in, 2 out]
        n166 = property on="Final Line" class="DigNum (strict)"("DisabledEnum"=w378) -> ()  [unwired: 2 in, 2 out]
        n167 = property on="Final Column" class="DigNum (strict)"("DisabledEnum"=w378) -> ()  [unwired: 2 in, 2 out]
        n168 = flat-sequence {
          tunnel: w383 -> [w401]
          tunnel: w384 -> [w402]
          tunnel: [w402] -> w382
          tunnel: [w401] -> w381
          frame #0 {
            w395 = cluster{dbl, dbl} {0.0, 0.0}
            n169 = local read "Initial Cloumn"() -> (w394:u16)
            n170 = local read "Final Column"() -> (w392:u16)
            n171 = local read "Final Line"() -> (w393:u16)
            n172 = local read "Final Line"() -> (w391:u16)
            n173 = Bundle(cluster=w395, w394, w393) -> (w400:cluster{dbl, dbl})
            n174 = Bundle(cluster=w395, w394, w391) -> (w399:cluster{dbl, dbl})
            n175 = Bundle(cluster=w395, w392, w391) -> (w398:cluster{dbl, dbl})
            n176 = Bundle(cluster=w395, w392, w393) -> (w397:cluster{dbl, dbl})
            n177 = Bundle(cluster=w395, w394, w393) -> (w396:cluster{dbl, dbl})
            n178 = Build Array(w400, w399, w398, w397, w396) -> ()  [unwired: 1 out]
          }
        }
      }
      event "Acquisition Mode": Value Change {
        n179 = event-data() -> ("NewVal"=w404:u16)  [unwired: 1 in]
        n180 = case shown="1, Default" w404 {
          tunnel: [T9."Enabled" ("Disabled") T9."Disabled and Grayed Out" ("Disabled")] -> w403
          frame 3 {
          }
          frame 1, Default {
          }
        }
        n181 = property on="#frames" class="DigNum (strict)"("DisabledEnum"=w403) -> ()  [unwired: 2 in, 2 out]
      }
      event "calib wheel": Value Change {
        n182 = event-data() -> ()  [unwired: 1 in, 1 out]
        n183 = call-dynamic "Read S4ICS.lvclass.vi"("error in (no error)"=w424, "S4GEI in"=w425) -> ("error out"=w422:errorcluster, "S4ICS.lvclass"=w423:refnum<class "S4ICS.lvclass">, "S4GEI out"=w417:refnum<class "S4GEI.lvclass">)  [unwired: 7 in]
        n184 = call-dynamic "Read polarimeitrc config.vi"("error in (no error)"=w422, "S4ICS in"=w423) -> ("error out"=w418:errorcluster, "polarimeitrc config"=w421:T17, "S4ICS out"=w419:refnum<class "S4ICS.lvclass">)  [unwired: 7 in]
        n185 = Bundle By Name(cluster=w421, "calib wheel"="calib wheel") -> (w420:T17)
        n186 = call-dynamic "Write polarimetric config.vi"("error in (no error)"=w418, "polarimeitrc config"=w420, "S4ICS in"=w419) -> ("error out"=w415:errorcluster, "S4ICS out"=w416:refnum<class "S4ICS.lvclass">)  [unwired: 7 in]
        n187 = call-dynamic "Write S4ICS.lvclass.vi"("error in (no error)"=w415, "S4ICS.lvclass"=w416, "S4GEI in"=w417) -> ("error out"=w414:errorcluster, "S4GEI out"=w413:refnum<class "S4GEI.lvclass">)  [unwired: 7 in]
        n188 = call "Write State.vi"("error in (no error)"=w414, "State"="SET_CALW", "SPARC4_GEI in"=w413) -> ("error out"=w411:errorcluster, "SPARC4_GEI out"=w412:refnum<class "S4GEI.lvclass">)  [unwired: 7 in]
      }
      event "waveplate": Value Change {
        n189 = event-data() -> ("NewVal"=w426:u16)  [unwired: 1 in]
        n190 = call-dynamic "Read S4ICS.lvclass.vi"("error in (no error)"=w443, "S4GEI in"=w444) -> ("error out"=w441:errorcluster, "S4ICS.lvclass"=w442:refnum<class "S4ICS.lvclass">, "S4GEI out"=w436:refnum<class "S4GEI.lvclass">)  [unwired: 7 in]
        n191 = call-dynamic "Read polarimeitrc config.vi"("error in (no error)"=w441, "S4ICS in"=w442) -> ("error out"=w437:errorcluster, "polarimeitrc config"=w440:T17, "S4ICS out"=w438:refnum<class "S4ICS.lvclass">)  [unwired: 7 in]
        n192 = Bundle By Name(cluster=w440, "waveplate"="waveplate") -> (w439:T17)
        n193 = call-dynamic "Write polarimetric config.vi"("error in (no error)"=w437, "polarimeitrc config"=w439, "S4ICS in"=w438) -> ("error out"=w434:errorcluster, "S4ICS out"=w435:refnum<class "S4ICS.lvclass">)  [unwired: 7 in]
        n194 = call-dynamic "Write S4ICS.lvclass.vi"("error in (no error)"=w434, "S4ICS.lvclass"=w435, "S4GEI in"=w436) -> ("error out"=w432:errorcluster, "S4GEI out"=w433:refnum<class "S4GEI.lvclass">)  [unwired: 7 in]
        n195 = call "Write State.vi"("error in (no error)"=w432, "State"="SET_WPSEL", "SPARC4_GEI in"=w433) -> ("error out"=w429:errorcluster, "SPARC4_GEI out"=w427:refnum<class "S4GEI.lvclass">)  [unwired: 7 in]
        n196 = case shown="2" w426 {
          tunnel: w429 -> [w445 w447]
          tunnel: [w445 w447] -> w428
          frame 0, Default {
          }
          frame 2 {
            n197 = local write "waveplate positions"(T2 {"WP 1"=TRUE, "WP 2"=FALSE, "WP 3"=FALSE, "WP 4"=FALSE, "WP 5"=FALSE, "WP 6"=FALSE, "WP 7"=FALSE, "WP 8"=FALSE, "WP 9"=FALSE, "WP 10"=FALSE, "WP 11"=FALSE, "WP 12"=FALSE, "WP 13"=FALSE, "WP 14"=FALSE, "WP 15"=FALSE, "WP 16"=FALSE} ("waveplate positions")) -> ()
          }
        }
      }
      event "wppos presents": Value Change {
        n198 = event-data() -> ()  [unwired: 1 in, 1 out]
        n199 = local read "waveplate positions"() -> (w448:T2)
        n200 = case shown="0, Default" "wppos presents" {
          tunnel: [T11 {"WP 1"=TRUE, "WP 2"=FALSE, "WP 3"=FALSE, "WP 4"=FALSE, "WP 5"=FALSE, "WP 6"=FALSE, "WP 9"=FALSE, "WP 8"=FALSE, "WP 7"=FALSE, "WP 10"=FALSE, "WP 11"=FALSE, "WP 12"=FALSE, "WP 13"=FALSE, "WP 14"=FALSE, "WP 15"=FALSE, "WP 16"=FALSE} ("waveplate positions") T11 {"WP 1"=TRUE, "WP 2"=TRUE, "WP 3"=TRUE, "WP 4"=TRUE, "WP 5"=TRUE, "WP 6"=TRUE, "WP 9"=TRUE, "WP 8"=TRUE, "WP 7"=TRUE, "WP 10"=TRUE, "WP 11"=TRUE, "WP 12"=TRUE, "WP 13"=TRUE, "WP 14"=TRUE, "WP 15"=TRUE, "WP 16"=TRUE} ("waveplate positions") T11 {"WP 1"=TRUE, "WP 2"=TRUE, "WP 3"=TRUE, "WP 4"=TRUE, "WP 5"=TRUE, "WP 6"=TRUE, "WP 9"=TRUE, "WP 8"=TRUE, "WP 7"=FALSE, "WP 10"=FALSE, "WP 11"=FALSE, "WP 12"=FALSE, "WP 13"=FALSE, "WP 14"=FALSE, "WP 15"=FALSE, "WP 16"=FALSE} ("waveplate positions") T11 {"WP 1"=TRUE, "WP 2"=TRUE, "WP 3"=TRUE, "WP 4"=TRUE, "WP 5"=FALSE, "WP 6"=FALSE, "WP 9"=FALSE, "WP 8"=FALSE, "WP 7"=FALSE, "WP 10"=FALSE, "WP 11"=FALSE, "WP 12"=FALSE, "WP 13"=FALSE, "WP 14"=FALSE, "WP 15"=FALSE, "WP 16"=FALSE} ("waveplate positions") T11 {"WP 1"=TRUE, "WP 2"=TRUE, "WP 3"=TRUE, "WP 4"=TRUE, "WP 5"=FALSE, "WP 6"=FALSE, "WP 9"=FALSE, "WP 8"=FALSE, "WP 7"=TRUE, "WP 10"=TRUE, "WP 11"=TRUE, "WP 12"=TRUE, "WP 13"=FALSE, "WP 14"=FALSE, "WP 15"=FALSE, "WP 16"=FALSE} ("waveplate positions") w458] -> w449
          tunnel: w448 -> [_ _ _ _ _ w458]
          frame 0, Default {
          }
          frame 1 {
          }
          frame 2 {
          }
          frame 3 {
          }
          frame 4 {
          }
          frame 5 {
          }
        }
        n201 = local write "waveplate positions"(w449) -> ()
      }
      event "Cooler": Value Change {
        n202 = event-data() -> ()  [unwired: 1 in, 1 out]
        n203 = call "Read Channel lvclass.vi"("error in (no error)"=w474, "SPARC4_GUI in"=w475) -> ("error out"=w481:errorcluster, "Channel.lvclass"=w477:refnum<class "Channel.lvclass">, "SPARC4_GUI out"=w480:refnum<class "S4GEI.lvclass">)  [unwired: 7 in]
        n204 = call-dynamic "Read Camera.lvclass.vi"("error in (no error)"=w481, "Channel in"=w477) -> ("error out"=w472:errorcluster, "Camera.lvclass"=w473:refnum<class "Camera.lvclass">, "Channel out"=w476:refnum<class "Channel.lvclass">)  [unwired: 7 in]
        n205 = Boolean To (0,1)(Boolean="Cooler") -> (0, 1=w464:i16)
        n206 = call-dynamic "Read SET parameters.vi"("error in (no error)"=w472, "Camera in"=w473) -> ("error out"=w468:errorcluster, "SET parameters"=w467:T14, "Camera out"=w469:refnum<class "Camera.lvclass">)  [unwired: 7 in]
        n207 = Bundle By Name(cluster=w467, "COOLER_POWER_STATUS"=w464) -> (w466:T14)
        n208 = call-dynamic "Write SET parameters.vi"("error in (no error)"=w468, "SET parameters"=w466, "Camera in"=w469) -> ("error out"=w470:errorcluster, "Camera out"=w471:refnum<class "Camera.lvclass">)  [unwired: 7 in]
        n209 = call-dynamic "Write Camera.lvclass.vi"("error in (no error)"=w470, "Camera.lvclass"=w471, "Channel in"=w476) -> ("error out"=w479:errorcluster, "Channel out"=w478:refnum<class "Channel.lvclass">)  [unwired: 7 in]
        n210 = call "Write Channel lvclass.vi"("error in (no error)"=w479, "Channel.lvclass"=w478, "SPARC4_GUI in"=w480) -> ("error out"=w462:errorcluster, "SPARC4_GUI out"=w463:refnum<class "S4GEI.lvclass">)  [unwired: 7 in]
        n211 = call "write request state.vi"("error in (no error)"=w462, "State"="SET_COOLER", "S4GEI in"=w463) -> ("error out"=w460:errorcluster, "S4GEI out"=w461:refnum<class "S4GEI.lvclass">)  [unwired: 7 in]
      }
      event "Temp": Value Change {
        n212 = event-data() -> ()  [unwired: 1 in, 6 out]
        n213 = call "Read Channel lvclass.vi"("error in (no error)"=w496, "SPARC4_GUI in"=w497) -> ("error out"=w503:errorcluster, "Channel.lvclass"=w499:refnum<class "Channel.lvclass">, "SPARC4_GUI out"=w502:refnum<class "S4GEI.lvclass">)  [unwired: 7 in]
        n214 = call-dynamic "Read Camera.lvclass.vi"("error in (no error)"=w503, "Channel in"=w499) -> ("error out"=w494:errorcluster, "Camera.lvclass"=w495:refnum<class "Camera.lvclass">, "Channel out"=w498:refnum<class "Channel.lvclass">)  [unwired: 7 in]
        n215 = call-dynamic "Read SET parameters.vi"("error in (no error)"=w494, "Camera in"=w495) -> ("error out"=w490:errorcluster, "SET parameters"=w489:T14, "Camera out"=w491:refnum<class "Camera.lvclass">)  [unwired: 7 in]
        n216 = Bundle By Name(cluster=w489, "TEMP"="Temp") -> (w488:T14)
        n217 = call-dynamic "Write SET parameters.vi"("error in (no error)"=w490, "SET parameters"=w488, "Camera in"=w491) -> ("error out"=w492:errorcluster, "Camera out"=w493:refnum<class "Camera.lvclass">)  [unwired: 7 in]
        n218 = call-dynamic "Write Camera.lvclass.vi"("error in (no error)"=w492, "Camera.lvclass"=w493, "Channel in"=w498) -> ("error out"=w501:errorcluster, "Channel out"=w500:refnum<class "Channel.lvclass">)  [unwired: 7 in]
        n219 = call "Write Channel lvclass.vi"("error in (no error)"=w501, "Channel.lvclass"=w500, "SPARC4_GUI in"=w502) -> ("error out"=w486:errorcluster, "SPARC4_GUI out"=w487:refnum<class "S4GEI.lvclass">)  [unwired: 7 in]
        n220 = call "write request state.vi"("error in (no error)"=w486, "State"="SET_TEMP", "S4GEI in"=w487) -> ("error out"=w484:errorcluster, "S4GEI out"=w485:refnum<class "S4GEI.lvclass">)  [unwired: 7 in]
      }
      event "auto adv mode": Value Change {
        n221 = event-data() -> ()  [unwired: 1 in, 6 out]
        n222 = call "Read Channel lvclass.vi"("error in (no error)"=w513, "SPARC4_GUI in"=w514) -> ("error out"=w507:errorcluster, "Channel.lvclass"=w508:refnum<class "Channel.lvclass">, "SPARC4_GUI out"=w512:refnum<class "S4GEI.lvclass">)  [unwired: 7 in]
        n223 = call "Write automatic adv mode.vi"("error in (no error)"=w507, "automatic adv mode"="auto adv mode", "Channel in"=w508) -> ("error out"=w506:errorcluster, "Channel out"=w509:refnum<class "Channel.lvclass">)  [unwired: 7 in]
        n224 = call "Write Channel lvclass.vi"("error in (no error)"=w506, "Channel.lvclass"=w509, "SPARC4_GUI in"=w512) -> ("error out"=w510:errorcluster, "SPARC4_GUI out"=w511:refnum<class "S4GEI.lvclass">)  [unwired: 7 in]
        n225 = call "write request state.vi"("error in (no error)"=w510, "State"="AUTO_ADV_MODE", "S4GEI in"=w511) -> ("error out"=w515:errorcluster, "S4GEI out"=w516:refnum<class "S4GEI.lvclass">)  [unwired: 7 in]
      }
    }
    n226 = Unbundle By Name(w14) -> ("status"=w19:bool)
    n227 = Or(x=w19, y="Stop Application") -> (x .or. y?=w20:bool)
  }
  n228 = Unbundle By Name(w10) -> ("source"=→"Error Message":string)
  n229 = call <vilib>:"Clear Errors.vi"("error in (no error)"=w10) -> ("error out"=w9:errorcluster)  [unwired: 5 in, 1 out]
  n230 = call "End.vi"("error in (no error)"=w9, "SPARC4_GUI in"=w12) -> ("SPARC4_GUI out"=w13:refnum<class "S4GEI.lvclass">)  [unwired: 8 in, 1 out]
  n231 = flat-sequence {
    tunnel: w13 -> [_]
    frame #0 {
      w519 = T7 {"mode"="", "condition"="", "position"="", "pos_name"="", "pos_id"=""} ("WPROT status")
      w520 = 1
      w521 = u16 2 items=["L/4"=1, "OFF"=2, "L/2"=3] ("current waveplate")
      w522 = u16 3 items=["PINHOLE"=1, "POLARIZER"=2, "OFF"=3, "SHUTTER"=4, "DEPOLARIZER"=5] ("current calw")
      w523 = u16 3 items=["PINHOLE"=1, "POLARIZER"=2, "OFF"=3, "SHUTTER"=4, "DEPOLARIZER"=5] ("calib wheel")
      w524 = u16 2 items=["L/4"=1, "OFF"=2, "L/2"=3] ("waveplate")
      w527 = ""
      w528 = FALSE ("analyser status")
      w532 = u16 0 items=["Clear", "All positions", "First 8 positions", "First 4 positions", "1-4 & 9-12", "Customized"] ("wppos presents")
      w533 = FALSE ("pol mode")
      w540 = u16 1 items=["U"=1, "B"=2, "V"=3, "R"=4, "I"=5, "Clear"=6] ("Current filter")
      w551 = u16 0 items=["Internal", "External", "N/A", "N/A", "N/A", "N/A", "External Start", "External Exposure (Bulb)", "N/A", "External FVB EM", "Software", "N/A", "External Charge Shifting"] ("Trigger Mode")
      w552 = u16 4 items=["Full Vertical Binning", "Multi-Track", "Random-Track", "Single-Track", "Image"] ("Read Mode")
      w553 = u16 3 items=["Reserved", "Single Scan", "Accumulate", "Kinetic", "Fast Kinetic", "Run till abort", "Reserved", "Reserved", "Reserved", "Time Delayed Integration"] ("Acquisition Mode")
      w558 = u16 0 items=["TTL Low", "TTL High"] ("Shutter TTL")
      w560 = u8 0 items=["  1 MHz", "0.1 MHz"] ("Readout Rate")
      w562 = u8 2 items=["Fully Auto", "OPEN", "CLOSED"] ("Shutter Mode")
      w526 = "" ("Command:")
      w564 = u16 1024 ("Final Line")
      w563 = u16 1 ("Initial Cloumn")
      w567 = u8 0 items=["Gain 1", "Gain 2"] ("Pre-amp gain")
      w568 = u8 1 items=["Electron Multiplying", "Conventional"] ("EM Mode")
      n232 = local write "#frames"(w520) -> ()
      n233 = local write "#cycles"(w520) -> ()
      n234 = property on="Cycles done" class="Slide (strict)"("Scale.Maximum"=1.0 ("Scale.Range:Maximum")) -> ()  [unwired: 2 in, 2 out]
      n235 = property on="Frames done" class="Slide (strict)"("Scale.Maximum"=1.0 ("Scale.Range:Maximum")) -> ()  [unwired: 2 in, 2 out]
      n236 = local write "WPROT status"(w519) -> ()
      n237 = local write "GFOC status"(w519) -> ()
      n238 = local write "GMIR status"(w519) -> ()
      n239 = local write "ASEL status"(w519) -> ()
      n240 = local write "CALW status"(w519) -> ()
      n241 = local write "WPSEL status"(w519) -> ()
      n242 = property on="Sequences done" class="Slide (strict)"("Scale.Maximum"=1.0 ("Scale.Range:Maximum")) -> ()  [unwired: 2 in, 2 out]
      n243 = local write "CCD status"(T20 {"Cycles done"=1, "Sequences done"=1, "Frames done"=1, "CCD Status"="", "Exposing"=FALSE, "Last image"="", "temp"=0, "serial n"=0, "texp"=0.0, "used disk"=0, "Power"=FALSE, "ACS mode"=FALSE} ("CCD status")) -> ()
      n244 = property on="temp" class="DigNum (strict)"("NumText.BGColor"=u32 12369084) -> ()  [unwired: 2 in, 2 out]
      n245 = local write "phot mode"(w533) -> ()
      n246 = property on="Sequences done" class="Slide (strict)"("Scale.Maximum"=1.0 ("Scale.Range:Maximum"), "Scale.Minimum"=0.0 ("Scale.Range:Minimum")) -> ()  [unwired: 2 in, 2 out]
      n247 = local write "pol mode"(w533) -> ()
      n248 = local write "Command:"(w526) -> ()
      n249 = local write "observer"(w526) -> ()
      n250 = local write "projid"(w526) -> ()
      n251 = local write "file name suffix"(w527) -> ()
      n252 = local write "object name"(w527) -> ()
      n253 = local write "comment"(w527) -> ()
      n254 = property on="acs mode" class="Bool (strict)"("Colors [4]"=cluster{u32, u32}[] [{1985280, 1985280}, {1985280, 1985280}, {6618880, 6618880}]) -> ()  [unwired: 2 in, 2 out]
      n255 = local write "Acquisition configuration 6"(T22 {"Select"=FALSE, "Exp Time"=1, "#Frames"=1, "Sufix"="", "Filter"=6} ("Acquisition configuration 6")) -> ()
      n256 = local write "Acquisition configuration 5"(T22 {"Select"=FALSE, "Exp Time"=1, "#Frames"=1, "Sufix"="", "Filter"=5} ("Acquisition configuration 5")) -> ()
      n257 = local write "Acquisition configuration 4"(T22 {"Select"=FALSE, "Exp Time"=1, "#Frames"=1, "Sufix"="", "Filter"=4} ("Acquisition configuration 4")) -> ()
      n258 = local write "Acquisition configuration 3"(T22 {"Select"=FALSE, "Exp Time"=1, "#Frames"=1, "Sufix"="", "Filter"=3} ("Acquisition configuration 3")) -> ()
      n259 = local write "Acquisition configuration 2"(T22 {"Select"=FALSE, "Exp Time"=1, "#Frames"=1, "Sufix"="", "Filter"=2} ("Acquisition configuration 2")) -> ()
      n260 = local write "Acquisition configuration"(T22 {"Select"=FALSE, "Exp Time"=1, "#Frames"=1, "Sufix"="", "Filter"=1} ("Acquisition configuration")) -> ()
      n261 = local write "Number of iterations"(u16 1 ("Number of iterations")) -> ()
      n262 = local write "Current filter"(w540) -> ()
      n263 = local write "Iterations Done"(u8 0 ("Iterations Done")) -> ()
      n264 = local write "wppos presents"(w532) -> ()
      n265 = local write "waveplate"(w524) -> ()
      n266 = local write "calib wheel"(w523) -> ()
      n267 = local write "waveplate positions"(T2 {"WP 1"=TRUE, "WP 2"=FALSE, "WP 3"=FALSE, "WP 4"=FALSE, "WP 5"=FALSE, "WP 6"=FALSE, "WP 7"=FALSE, "WP 8"=FALSE, "WP 9"=FALSE, "WP 10"=FALSE, "WP 11"=FALSE, "WP 12"=FALSE, "WP 13"=FALSE, "WP 14"=FALSE, "WP 15"=FALSE, "WP 16"=FALSE} ("waveplate positions")) -> ()
      n268 = local write "current calw"(w522) -> ()
      n269 = local write "current waveplate"(w521) -> ()
      n270 = local write "analyser status"(FALSE ("analyser status")) -> ()
      n271 = local write "preset modes"(T21 {"object"=FALSE, "test"=FALSE, "zero"=FALSE, "dark"=FALSE, "sflat"=FALSE, "dflat"=FALSE, "focus"=FALSE, "led object"=FALSE, "led test"=FALSE, "led zero"=FALSE, "led dark"=FALSE, "led sflat"=FALSE, "led dflat"=FALSE, "led foc"=FALSE} ("preset modes")) -> ()
      n272 = local write "start exp"(w528) -> ()
      n273 = local write "Stop Acquisition"(w528) -> ()
      n274 = local write "Abort Acquisition"(w528) -> ()
      n275 = local write "Pause acquisition"(w528) -> ()
      n276 = local write "current wppos"(T2 {"WP 1"=FALSE, "WP 2"=FALSE, "WP 3"=FALSE, "WP 4"=FALSE, "WP 5"=FALSE, "WP 6"=FALSE, "WP 7"=FALSE, "WP 8"=FALSE, "WP 9"=FALSE, "WP 10"=FALSE, "WP 11"=FALSE, "WP 12"=FALSE, "WP 13"=FALSE, "WP 14"=FALSE, "WP 15"=FALSE, "WP 16"=FALSE} ("current wppos")) -> ()
      n277 = local write "Frame Tansfer"(TRUE ("Frame Tansfer")) -> ()
      n278 = local write "Shutter TTL"(w558) -> ()
      n279 = local write "Shutter Time"(u16 50 ("Shutter Time")) -> ()
      n280 = local write "Vertical Shift Speed"(u16 3 ("Vertical Shift Speed")) -> ()
      n281 = local write "AD Channel"(u16 0 ("AD Channel")) -> ()
      n282 = local write "Vertical Clock Voltagem"(u16 0 ("Vertical Clock Voltagem")) -> ()
      n283 = local write "Acquisition Mode"(w553) -> ()
      n284 = local write "Read Mode"(w552) -> ()
      n285 = local write "Trigger Mode"(w551) -> ()
      n286 = property on="Readout Rate" class="Ring (strict)"("Strings []"=string[] ["1 MHz", "0.1 MHz"]) -> ()  [unwired: 2 in, 2 out]
      n287 = local write "Shutter Mode"(w562) -> ()
      n288 = local write "EM Gain"(u16 2 ("EM Gain")) -> ()
      n289 = local write "EM Mode"(w568) -> ()
      n290 = local write "Readout Rate"(w560) -> ()
      n291 = local write "Pre-amp gain"(w567) -> ()
      n292 = local write "Sub Image"(T5."1024 x 1024" ("Sub Image")) -> ()
      n293 = local write "Initial Line"(u16 1 ("Initial Line")) -> ()
      n294 = local write "Final Line"(w564) -> ()
      n295 = local write "Final Column"(w564) -> ()
      n296 = local write "Initial Cloumn"(w563) -> ()
      n297 = local write "Binning"(w563) -> ()
      n298 = property on="#frames" class="DigNum (strict)"("DisabledEnum"=T9."Enabled" ("Disabled")) -> ()  [unwired: 2 in, 2 out]
      n299 = property on="EM Gain" class="DigNum (strict)"("DisabledEnum"=T9."Disabled and Grayed Out" ("Disabled")) -> ()  [unwired: 2 in, 2 out]
    }
  }
